vi "Omniax_mDrive_XYZR_2017APXNoBK.vi"() -> ()   [LabVIEW 2015]
uses:
  <vilib>/Utility/file.llb/Read From Spreadsheet File (I64).vi
  <vilib>/Utility/file.llb/Read From Spreadsheet File (string).vi
  <vilib>/Instr/_visa.llb/VISA Configure Serial Port (Instr).vi
  <vilib>/Utility/file.llb/Write To Spreadsheet File (I64).vi
  <vilib>/Utility/file.llb/Write To Spreadsheet File (string).vi
panel:
  out "Boolean 3":bool
  out "Boolean 2":bool
  out "Boolean":bool
  out "read buffer":string
  out "sum":dbl
  in  "Open?":bool
  out "Z max step":i32
  in  "V5 position 15360000":i32
  out "NC":bool
  out "R Velocity MVdeg/sec":dbl format="%.3f"
  out "R Position MV deg":dbl
  out "Z Velocity MV mm/sec":dbl format="%.3f"
  out "Z Position MV mm":dbl
  out "Y Velocity MV mm/sec":dbl format="%.3f"
  out "Y Position MV mm":dbl
  out "X Velocity MV mm/sec":dbl format="%.3f"
  out "X Position MV mm":dbl
  out "Presets":i32[][](array[numeric])
  in  "stop":bool
  in  "Tab Control 3":enum32{"Status", "Reset"}(tab)
  out "APX:Y_LIM":bool
  out "APX:MY_MVG":bool
  out "APX:X_LIM":bool
  out "APX:MX_MVG":bool
  out "APX:MZ_LIM":bool
  out "APX:MZ_MVG":bool
  out "APX:MR_LIM":bool
  out "APX:MR_MVG":bool
  out "APX:MX_RDY":bool
  out "APX:MY_RDY":bool
  out "APX:MZ_RDY":bool
  out "APX:MR_RDY":bool
  in  "Reset Y Position mm":dbl
  out "Reset Y Motor Steps":i32
  in  "Reset X Position mm":dbl
  out "Reset X Motor Steps":i32
  in  "Reset Z Position mm":dbl
  out "Reset Z Motor Steps":i32
  in  "Reset R Position deg":dbl
  out "Reset R Motor Steps":i32
  in  "Reset":bool
  in  "Tab Control":enum32{"mm", "preset", "step"}(tab)
  in  "APX:MX_RQ":dbl min=-1.28 max=1.28
  in  "APX:MX_VLC_RQ":dbl min=0.0 max=0.4 step=0.1
  in  "APX:MY_RQ":dbl min=-1.5 max=1.0
  in  "APX:MY_VLC_RQ":dbl min=0.0 max=0.4 step=0.1
  in  "APX:MZ_RQ":dbl=10.0 min=10.0 max=355.8 step=0.1
  in  "APX:MZ_VLC_RQ":dbl=0.20000000000000015 min=0.1 max=0.8 step=0.1
  in  "APX:MR_RQ":dbl
  in  "APX:MR_VLC_RQ":dbl
  in  "Add Button":bool
  in  "String":string
  in  "Delete Button":bool
  in  "Preset positions":i32(ring) items=["ZERO", "Default", "CDOSE", "QMS", "test", "test2", "test3", "yag position", "Sample Long Edge  ", "SPUTTER POS"]
  in  "Set Button":bool
  in  "X Velocity SP step/sec":i32 min=1 max=128000
  in  "Y Velocity SP step/sec":i32 min=1 max=128000
  in  "Z Velocity SP step/sec":i32 min=1 max=204800
  in  "R Velocity SP step/sec":i32 min=1 max=10000
  in  "Y Step SP":i32=-20000 min=-2304000 max=2304000 step=500
  in  "X Step SP":i32=-20000 min=-2304000 max=2304000 step=500
  in  "Z Step SP":i32=-20000 min=0 max=102400000 step=500
  in  "R Step SP":i32=-20000 min=-6144000 max=6144000 step=500
  out "X Step PV":i32 max=2000
  out "Y Step PV":i32 max=2000
  out "Z Step PV":i32 max=2000
  out "R Step PV":i32 max=2000
  in  "Clear ZY":bool
  out "R Backlash steps/sec":i32
  out "R Backlash":i32
  out "R Holding Current %":i32
  out "R Run Current %":i32
  out "R offset deg":dbl
  out "R deg/rev":dbl
  out "R steps/rev":u32
  out "R velocity PV step/sec":i32
  out "R MINPOS":i32=-94296
  out "R MAXPOS":i32=-34296
  out "R COM PORT":refnum<visa-resource-name>="COM5"
  out "APZ:MR_PV":dbl
  out "Z COM PORT":refnum<visa-resource-name>="COM5"
  out "Z Backlash steps/sec":i32
  out "Z Backlash":i32
  out "Z Holding Current %":i32
  out "Z Run Current %":i32
  out "Z offset mm":dbl
  out "Z mm/rev":dbl
  out "Z steps/rev":u32
  out "Z  velocity PV step/sec":i32
  out "Z MINPOS":i32=-94296
  out "Z MAXPOS":i32=-34296
  out "APX:MZ_PV":dbl
  out "APX:MX_PV":dbl
  out "X velocity PV step/sec":i32
  out "X Backlash steps/sec":i32
  out "X Backlash":i32
  out "X Holding Current %":i32
  out "X Run Current %":i32
  out "X offset mm":dbl
  out "X mm/rev":dbl
  out "X steps/rev":u32
  out "X MAXPOS":i32=-34296
  out "X MINPOS":i32=-94296
  out "X COM PORT":refnum<visa-resource-name>="COM5"
  out "Y Backlash steps/sec":i32
  out "Y Backlash":i32
  out "Y Holding Current %":i32
  out "Y Run Current %":i32
  out "APX:MY_PV":dbl
  out "Y offset mm":dbl
  out "Y mm/rev":dbl
  out "Y steps/rev":u32
  out "Y velocity PV step/sec":i32
  in  "APX:MXYZR_STOP":bool
  out "Y MINPOS":i32=-94296
  out "Y MAXPOS":i32=-34296
  out "Y COM PORT":refnum<visa-resource-name>="COM5"
  # "12-15"
  # "Current position"
  # "Goto position"
  # "MX"
  # "MY"
  # "MZ"
  # "MR"
  # "Preset position"
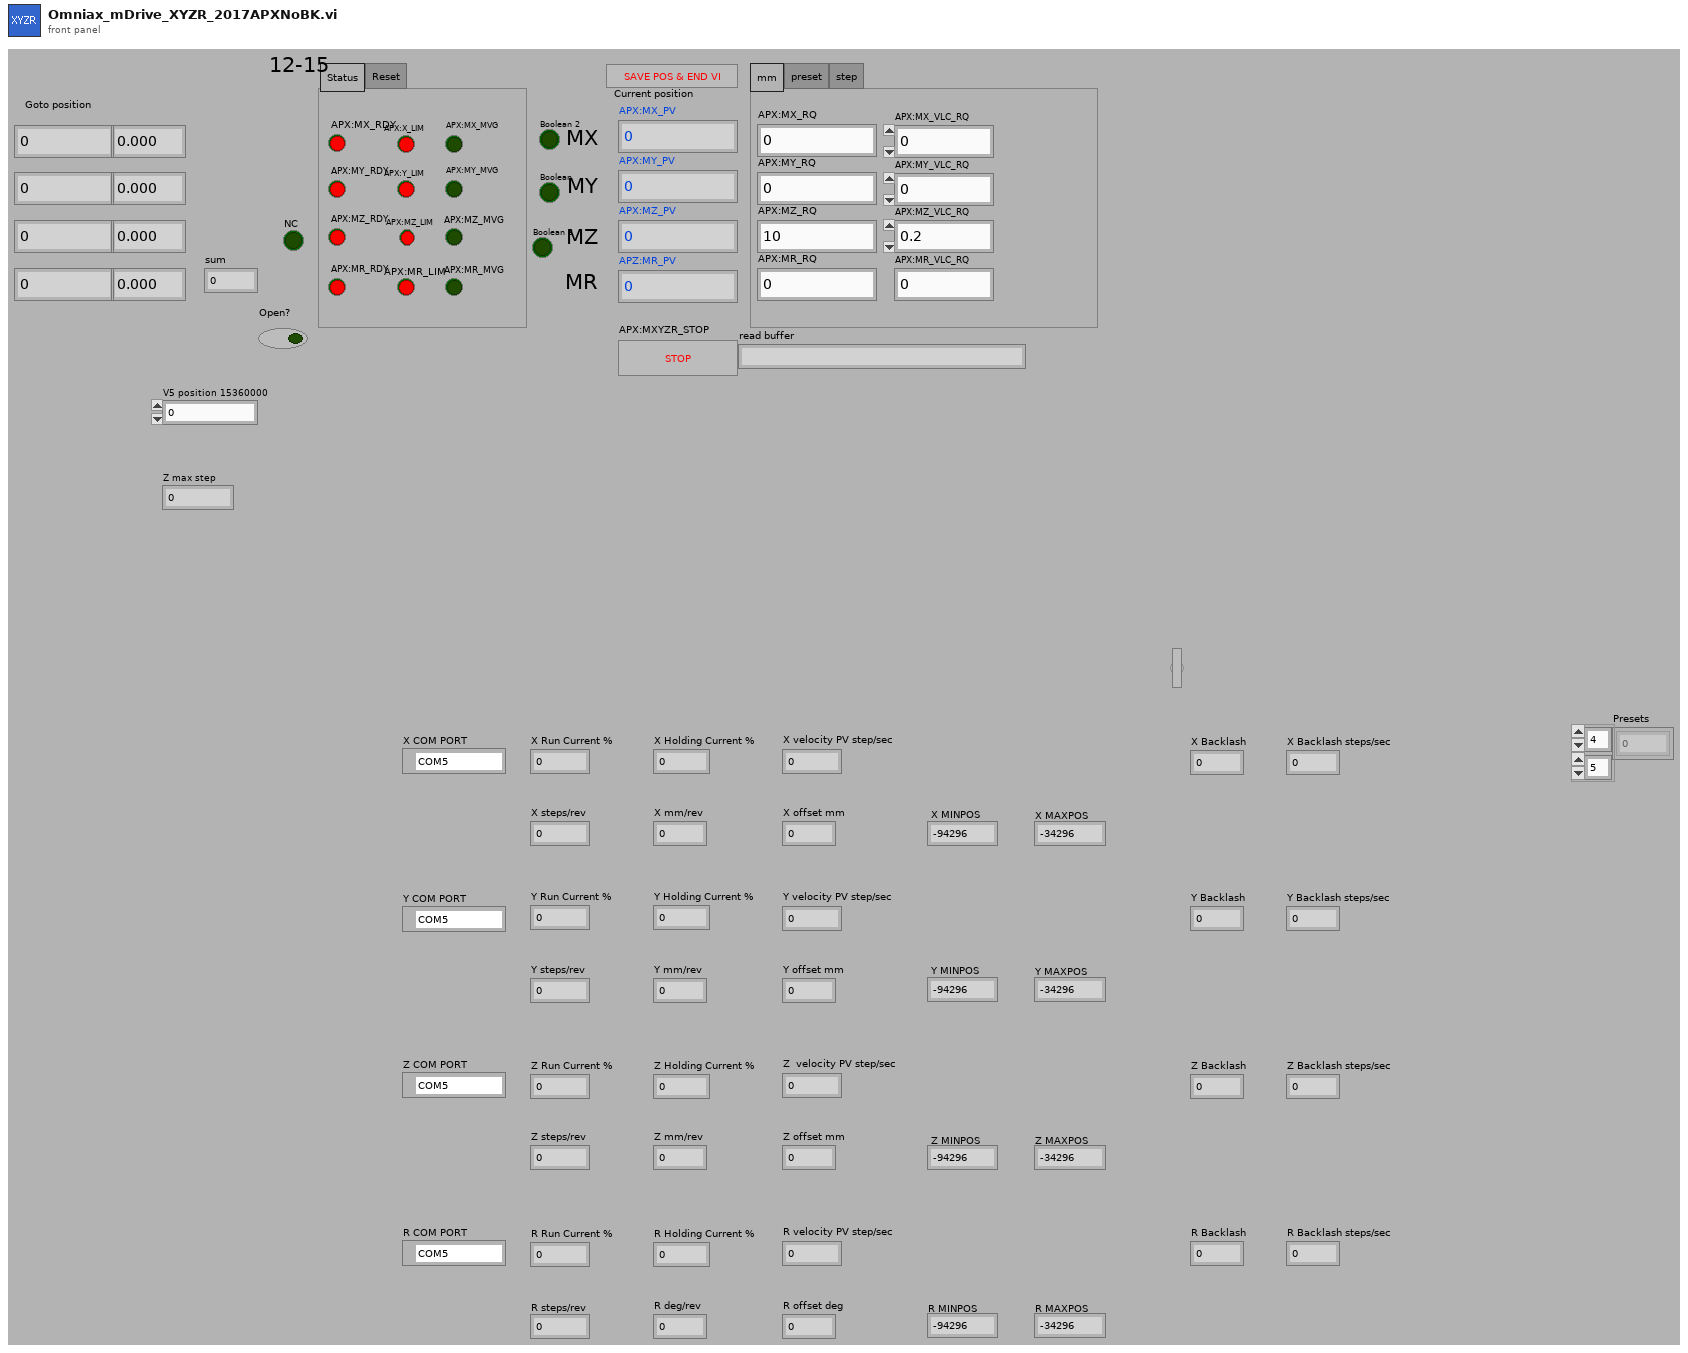
[diagram p1: front panel]
types:
  T1 = enum16{"Stop", "Reset", "Run Current", "Holding Current", "Accel Rate", "Decel Rate", "Move to Relative Position", "Move to Absolute Position", "Echo Mode", "Print Parameter", "Send String", "Microstep Resolution", "Set Current Position", "Max Velocity"}
  T2 = enum8{"Enabled", "Disabled", "Disabled and Grayed Out"}
  T3 = cluster{"first row[0]":i64, "first row[1]":i64, "first row[2]":i64, "first row[3]":i64, "first row[4]":i64, "first row[5]":i64, "first row[6]":i64, "first row[7]":i64, "first row[8]":i64}
  T4 = cluster{"Value[0]":i32, "Value[1]":i32, "Value[2]":i32, "Value[3]":i32, "Value[4]":i32, "Value[5]":i32, "Value[6]":i32, "Value[7]":i32, "Value[8]":i32}
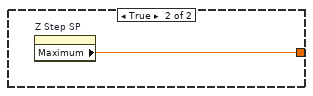
[diagram p9: hidden frame]
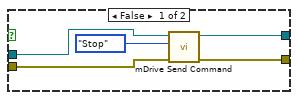
[diagram p15: hidden frame]
diagram:
  w2 = 0 ("dimension size")
  n1 = disable-structure shown="Disabled" {
    disable-tunnel: [w106 _] -> _
    disable-tunnel: [w105 _] -> _
    frame Disabled {
      n2 = call "DigitalIO_sub_V5_MON.vi"() -> ("CL"=w105:bool, "OP"=w106:bool)  [unwired: 8 in]
    }
    frame Enabled {
    }
  }
  n3 = disable-structure shown="Disabled" {
    frame Disabled {
      n4 = flat-sequence {
        frame #0 {
          w107 = FALSE ("Value (Signaling)")
          w110 = FALSE ("Value (Signaling)")
          w113 = FALSE ("Value (Signaling)")
          w114 = FALSE ("Value (Signaling)")
          "Z Backlash steps/sec" <- 25600 ("Z Backlash steps/sec")
          "Z Backlash" <- -51200 ("Z Backlash")
          "X Backlash steps/sec" <- 25600 ("Value (Signaling)")
          "X Backlash" <- 10240 ("Backlash2")
          "Y Backlash" <- -10240 ("Backlash2")
          "Y Backlash steps/sec" <- 25600 ("Value (Signaling)")
          "R Backlash steps/sec" <- 6400 ("R Backlash steps/sec")
          "R Backlash" <- -12800 ("R Backlash")
        }
      }
    }
    frame Enabled {
    }
  }
  n5 = flat-sequence {
    tunnel: [w120] -> w34
    tunnel: [w119] -> w33
    tunnel: [w132] -> w50
    tunnel: [w130] -> w48
    tunnel: w34 -> [w129]
    tunnel: w33 -> [w131]
    tunnel: w50 -> [w138]
    tunnel: [w139] -> w49
    tunnel: w48 -> [w135]
    tunnel: [w137] -> w47
    tunnel: [w148] -> w100
    tunnel: [w150] -> w98
    tunnel: w49 -> [w149]
    tunnel: w47 -> [w151]
    tunnel: w100 -> [w158]
    tunnel: [w157] -> w99
    tunnel: w98 -> [w155]
    tunnel: [w156] -> w97
    tunnel: [w168] -> w102
    tunnel: [w169] -> w101
    tunnel: w99 -> [w167]
    tunnel: w97 -> [w166]
    tunnel: w102 -> [w179]
    tunnel: w101 -> [w178]
    tunnel: [w181] -> w86
    tunnel: [w180] -> w85
    tunnel: [w175] -> w84
    tunnel: [w186] -> w103
    tunnel: [w187] -> w104
    tunnel: w86 -> [w187]
    tunnel: w85 -> [w186]
    tunnel: w84 -> [w182]
    frame #0 {
      w127 = refnum<visa-resource-name> "COM13" ("COM PORT")
      w125 = u16 0 items=["None", "XON/XOFF", "RTS/CTS", "XON/XOFF & RTS/CTS", "DTR/DSR", "XON/XOFF & DTR/DSR"] ("flow control (0:none)")
      w124 = u16 10 items=["1.0"=10, "1.5"=15, "2.0"=20] ("stop bits (10: 1 bit)")
      # "Stop bits"
      n6 = call-poly "VISA Configure Serial Port"("VISA resource name"=w127, "timeout (10sec)"=u32 10000, "baud rate (9600)"=u32 9600, "data bits (8)"=u16 8, "parity (0:none)"=enum16{"None", "Odd", "Even", "Mark", "Space"}."None", "stop bits (10: 1 bit)"=w124, "flow control (0:none)"=w125) -> ("VISA resource name out"=w120:refnum<visa-resource-name>, "error out"=w119:errorcluster)  [unwired: 7 in]
      "Y COM PORT" <- w127
    }
    frame #1 {
      n7 = VISA Flush I/O Buffer(VISA resource name=w129) -> (VISA resource name out=w128:refnum<visa-resource-name>)  [unwired: 2 in, 1 out]
      n8 = call "mDrive Send Command.vi"("error in (no error)"=w131, "Extra"="EM 2", "Command"=T1."Send String", "VISA resource name"=w128) -> ("error out"=w130:errorcluster, "VISA resource name out"=w132:refnum<visa-resource-name>)  [unwired: 3 in, 1 out]
    }
    frame #2 {
      n9 = Number To Decimal String(number=1000000) -> (decimal integer string=w140:string)  [unwired: 1 in]
      n10 = call "mDrive Send Command.vi"("error in (no error)"=w135, "Extra"=w140, "Command"=T1."Accel Rate", "VISA resource name"=w138) -> ("error out"=w136:errorcluster, "VISA resource name out"=w144:refnum<visa-resource-name>)  [unwired: 3 in, 1 out]
      n11 = call "mDrive Send Command.vi"("error in (no error)"=w136, "Extra"=w140, "Command"=T1."Decel Rate", "VISA resource name"=w144) -> ("error out"=w137:errorcluster, "VISA resource name out"=w139:refnum<visa-resource-name>)  [unwired: 3 in, 1 out]
    }
    frame #3 {
      # "Run Current %"
      n12 = property on="Y Run Current %" class="DigNum (strict)"() -> ("Value"=w146:i32)  [unwired: 2 in, 2 out]
      n13 = Number To Decimal String(number=w146) -> (decimal integer string=w147:string)  [unwired: 1 in]
      n14 = call "mDrive Send Command.vi"("error in (no error)"=w151, "Extra"=w147, "Command"=T1."Run Current", "VISA resource name"=w149) -> ("error out"=w150:errorcluster, "VISA resource name out"=w148:refnum<visa-resource-name>)  [unwired: 3 in, 1 out]
    }
    frame #4 {
      # "Holding Current %"
      n15 = property on="Y Holding Current %" class="DigNum (strict)"() -> ("Value"=w153:i32)  [unwired: 2 in, 2 out]
      n16 = Number To Decimal String(number=w153) -> (decimal integer string=w154:string)  [unwired: 1 in]
      n17 = call "mDrive Send Command.vi"("error in (no error)"=w155, "Extra"=w154, "Command"=T1."Holding Current", "VISA resource name"=w158) -> ("error out"=w156:errorcluster, "VISA resource name out"=w157:refnum<visa-resource-name>)  [unwired: 3 in, 1 out]
    }
    frame #5 {
      # "Velocity Max"
      n18 = property on="Y Velocity SP step/sec" class="DigNum (strict)"() -> ("Value"=w165:i32)  [unwired: 2 in, 2 out]
      n19 = Number To Decimal String(number=w165) -> (decimal integer string=w164:string)  [unwired: 1 in]
      n20 = call "mDrive Send Command.vi"("error in (no error)"=w166, "Extra"=w164, "Command"=T1."Max Velocity", "VISA resource name"=w167) -> ("error out"=w162:errorcluster, "VISA resource name out"=w172:refnum<visa-resource-name>)  [unwired: 3 in, 1 out]
      n21 = call "mDrive Send Command.vi"("error in (no error)"=w162, "Extra"="VM", "Command"=T1."Print Parameter", "VISA resource name"=w172) -> ("error out"=w169:errorcluster, "read buffer"=w170:string, "VISA resource name out"=w168:refnum<visa-resource-name>)  [unwired: 3 in]
      n22 = Decimal String To Number(string=w170, offset=0) -> (number=w163:i32)  [unwired: 1 in, 1 out]
      n23 = property on="Y scan velocity MV step/sec" class="DigNum (strict)"("Val(Sgnl)"=w163) -> ()  [unwired: 2 in, 2 out]
    }
    frame #6 {
      # "PRINT POSITION"
      n24 = call "mDrive Send Command.vi"("error in (no error)"=w178, "Extra"="P", "Command"=T1."Print Parameter", "VISA resource name"=w179) -> ("error out"=w180:errorcluster, "read buffer"=w177:string, "VISA resource name out"=w181:refnum<visa-resource-name>)  [unwired: 3 in]
      n25 = Decimal String To Number(string=w177, offset=0) -> (number=w175:i32)  [unwired: 1 in, 1 out]
    }
    frame #7 {
      w184 = -2304000 ("lower limit")
      w185 = 2304000 ("upper limit")
      n26 = property on="Y Step SP" class="DigNum (strict)"("Val(Sgnl)"=w182) -> ()  [unwired: 2 in, 2 out]
      n27 = property on="Y Step SP" class="DigNum (strict)"("Maximum"=w185) -> ()  [unwired: 2 in, 2 out]
      n28 = In Range and Coerce(upper limit=w185, x=w182, lower limit=w184) -> (In Range?=w183:bool)  [unwired: 1 out]
      n29 = property on="Y Step SP" class="DigNum (strict)"("Minimum"=w184) -> ()  [unwired: 2 in, 2 out]
      n30 = property on="APX:Y_LIM" class="Bool (strict)"("Val(Sgnl)"=w183) -> ()  [unwired: 2 in, 2 out]
      "Y MINPOS" <- w184
      "Y MAXPOS" <- w185
    }
  }
  n31 = flat-sequence {
    tunnel: [w189] -> w36
    tunnel: [w188] -> w35
    tunnel: [w197] -> w54
    tunnel: [w199] -> w52
    tunnel: w36 -> [w198]
    tunnel: w35 -> [w200]
    tunnel: w54 -> [w204]
    tunnel: [w205] -> w53
    tunnel: w52 -> [w203]
    tunnel: [w206] -> w51
    tunnel: [w217] -> w71
    tunnel: [w219] -> w70
    tunnel: w53 -> [w218]
    tunnel: w51 -> [w213]
    tunnel: w71 -> [w226]
    tunnel: [w225] -> w69
    tunnel: w70 -> [w223]
    tunnel: [w224] -> w68
    tunnel: [w236] -> w67
    tunnel: [w237] -> w66
    tunnel: w69 -> [w235]
    tunnel: w68 -> [w234]
    tunnel: w67 -> [w247]
    tunnel: w66 -> [w246]
    tunnel: [w249] -> w65
    tunnel: [w248] -> w64
    tunnel: [w243] -> w63
    tunnel: [w256] -> w59
    tunnel: [w257] -> w60
    tunnel: w65 -> [w257]
    tunnel: w64 -> [w256]
    tunnel: w63 -> [w254]
    frame #0 {
      w196 = refnum<visa-resource-name> "COM15" ("COM PORT")
      w194 = u16 0 items=["None", "XON/XOFF", "RTS/CTS", "XON/XOFF & RTS/CTS", "DTR/DSR", "XON/XOFF & DTR/DSR"] ("flow control (0:none)")
      w193 = u16 10 items=["1.0"=10, "1.5"=15, "2.0"=20] ("stop bits (10: 1 bit)")
      # "Stop bits"
      n32 = call-poly "VISA Configure Serial Port"("VISA resource name"=w196, "timeout (10sec)"=u32 10000, "baud rate (9600)"=u32 9600, "data bits (8)"=u16 8, "parity (0:none)"=enum16{"None", "Odd", "Even", "Mark", "Space"}."None", "stop bits (10: 1 bit)"=w193, "flow control (0:none)"=w194) -> ("VISA resource name out"=w189:refnum<visa-resource-name>, "error out"=w188:errorcluster)  [unwired: 7 in]
      "R COM PORT" <- w196
    }
    frame #1 {
      n33 = call "mDrive Send Command.vi"("error in (no error)"=w200, "Extra"="EM 2", "Command"=T1."Send String", "VISA resource name"=w198) -> ("error out"=w199:errorcluster, "VISA resource name out"=w197:refnum<visa-resource-name>)  [unwired: 3 in, 1 out]
    }
    frame #2 {
      # "pr=1000000"
      n34 = Number To Decimal String(number=100000) -> (decimal integer string=w208:string)  [unwired: 1 in]
      n35 = call "mDrive Send Command.vi"("error in (no error)"=w203, "Extra"=w208, "Command"=T1."Accel Rate", "VISA resource name"=w204) -> ("error out"=w207:errorcluster, "VISA resource name out"=w212:refnum<visa-resource-name>)  [unwired: 3 in, 1 out]
      n36 = call "mDrive Send Command.vi"("error in (no error)"=w207, "Extra"=w208, "Command"=T1."Decel Rate", "VISA resource name"=w212) -> ("error out"=w206:errorcluster, "VISA resource name out"=w205:refnum<visa-resource-name>)  [unwired: 3 in, 1 out]
    }
    frame #3 {
      # "Run Current %"
      n37 = property on="R Run Current %" class="DigNum (strict)"() -> ("Value"=w215:i32)  [unwired: 2 in, 2 out]
      n38 = Number To Decimal String(number=w215) -> (decimal integer string=w216:string)  [unwired: 1 in]
      n39 = call "mDrive Send Command.vi"("error in (no error)"=w213, "Extra"=w216, "Command"=T1."Run Current", "VISA resource name"=w218) -> ("error out"=w219:errorcluster, "VISA resource name out"=w217:refnum<visa-resource-name>)  [unwired: 3 in, 1 out]
    }
    frame #4 {
      # "Holding Current %"
      n40 = property on="R Holding Current %" class="DigNum (strict)"() -> ("Value"=w221:i32)  [unwired: 2 in, 2 out]
      n41 = Number To Decimal String(number=w221) -> (decimal integer string=w222:string)  [unwired: 1 in]
      n42 = call "mDrive Send Command.vi"("error in (no error)"=w223, "Extra"=w222, "Command"=T1."Holding Current", "VISA resource name"=w226) -> ("error out"=w224:errorcluster, "VISA resource name out"=w225:refnum<visa-resource-name>)  [unwired: 3 in, 1 out]
    }
    frame #5 {
      # "Print Velocity Max"
      # "Velocity Max"
      n43 = property on="R Velocity SP step/sec" class="DigNum (strict)"() -> ("Value"=w233:i32)  [unwired: 2 in, 2 out]
      n44 = Number To Decimal String(number=w233) -> (decimal integer string=w232:string)  [unwired: 1 in]
      n45 = call "mDrive Send Command.vi"("error in (no error)"=w234, "Extra"=w232, "Command"=T1."Max Velocity", "VISA resource name"=w235) -> ("error out"=w230:errorcluster, "VISA resource name out"=w240:refnum<visa-resource-name>)  [unwired: 3 in, 1 out]
      n46 = call "mDrive Send Command.vi"("error in (no error)"=w230, "Extra"="VM", "Command"=T1."Print Parameter", "VISA resource name"=w240) -> ("error out"=w237:errorcluster, "read buffer"=w238:string, "VISA resource name out"=w236:refnum<visa-resource-name>)  [unwired: 3 in]
      n47 = Decimal String To Number(string=w238, offset=0) -> (number=w231:i32)  [unwired: 1 in, 1 out]
      n48 = property on="R velocity PV step/sec" class="DigNum (strict)"("Val(Sgnl)"=w231) -> ()  [unwired: 2 in, 2 out]
    }
    frame #6 {
      # "PRINT POSITION"
      n49 = call "mDrive Send Command.vi"("error in (no error)"=w246, "Extra"="P", "Command"=T1."Print Parameter", "VISA resource name"=w247) -> ("error out"=w248:errorcluster, "read buffer"=w245:string, "VISA resource name out"=w249:refnum<visa-resource-name>)  [unwired: 3 in]
      n50 = Decimal String To Number(string=w245, offset=0) -> (number=w243:i32)  [unwired: 1 in, 1 out]
    }
    frame #7 {
      n51 = property on="R Step SP" class="DigNum (strict)"("Val(Sgnl)"=w254) -> ()  [unwired: 2 in, 2 out]
      n52 = property on="R Step SP" class="DigNum (strict)"() -> ("Maximum"=w253:dbl)  [unwired: 2 in, 2 out]
      n53 = property on="R Step SP" class="DigNum (strict)"() -> ("Minimum"=w252:dbl)  [unwired: 2 in, 2 out]
      n54 = To Long Integer(number=w253) -> (32bit integer=w250:i32)
      "R MAXPOS" <- w250
      n55 = To Long Integer(number=w252) -> (32bit integer=w251:i32)
      "R MINPOS" <- w251
      n56 = In Range and Coerce(upper limit=w250, x=w254, lower limit=w251) -> (In Range?=w255:bool)  [unwired: 1 out]
      n57 = property on="APX:MR_LIM" class="Bool (strict)"("Val(Sgnl)"=w255) -> ()  [unwired: 2 in, 2 out]
    }
  }
  n58 = flat-sequence {
    frame #0 {
      w263 = -3.0 ("R deg/rev")
      w261 = u32 51200 ("step/rev")
      w265 = 10000 ("Value (Signaling)")
      n59 = To Double Precision Float(number=w265) -> (double precision float=w267:dbl)
      n60 = To Double Precision Float(number=w261) -> (double precision float=w262:dbl)
      n61 = property on="R Velocity SP step/sec" class="DigNum (strict)"("Val(Sgnl)"=w265) -> ()  [unwired: 2 in, 2 out]
      n62 = property on="R Velocity SP step/sec" class="DigNum (strict)"("Minimum"=1.0 ("Data Entry Limits:Minimum")) -> ()  [unwired: 2 in, 2 out]
      n63 = Divide(x=w267, y=w262) -> (x/y=w266:dbl)
      n64 = property on="R Velocity SP step/sec" class="DigNum (strict)"("Maximum"=w267) -> ()  [unwired: 2 in, 2 out]
      n65 = Multiply(x=w266, y=w263) -> (x*y=w264:dbl)
      n66 = Absolute Value(x=w264) -> (abs(x)=w258:dbl)
      n67 = property on="APX:MR_VLC_RQ" class="DigNum (strict)"("Val(Sgnl)"=w258) -> ()  [unwired: 2 in, 2 out]
      "R offset deg" <- 0.0 ("R offset deg")
      "R deg/rev" <- w263
      "R steps/rev" <- w261
    }
  }
  n68 = flat-sequence {
    frame #0 {
      w269 = 0.2 ("Z mm/rev")
      w268 = u32 51200 ("step/rev")
      w270 = 204800 ("Value (Signaling)")
      n69 = To Double Precision Float(number=w270) -> (double precision float=w274:dbl)
      n70 = To Double Precision Float(number=w268) -> (double precision float=w273:dbl)
      n71 = property on="Z Velocity SP step/sec" class="DigNum (strict)"("Val(Sgnl)"=w270) -> ()  [unwired: 2 in, 2 out]
      n72 = property on="Z Velocity SP step/sec" class="DigNum (strict)"("Minimum"=1.0 ("Data Entry Limits:Minimum")) -> ()  [unwired: 2 in, 2 out]
      n73 = Divide(x=w274, y=w273) -> (x/y=w271:dbl)
      n74 = property on="Z Velocity SP step/sec" class="DigNum (strict)"("Maximum"=w274) -> ()  [unwired: 2 in, 2 out]
      n75 = Multiply(x=w271, y=w269) -> (x*y=w272:dbl)
      n76 = property on="APX:MZ_VLC_RQ" class="DigNum (strict)"("Val(Sgnl)"=w272) -> ()  [unwired: 2 in, 2 out]
      "Z offset mm" <- 0.0 ("Z offset mm")
      "Z mm/rev" <- w269
      "Z steps/rev" <- w268
    }
  }
  n77 = flat-sequence {
    frame #0 {
      "Z Holding Current %" <- 20 ("Z Holding Current %")
      "Z Run Current %" <- 40 ("Z Run Current %")
      "X Run Current %" <- 40 ("Run Current %")
      "X Holding Current %" <- 20 ("Holding Current %")
      "Y Run Current %" <- 40 ("Run Current %")
      "Y Holding Current %" <- 20 ("Holding Current %")
      "R Holding Current %" <- 15 ("R Holding Current %")
      "R Run Current %" <- 80 ("R Run Current %")
    }
  }
  n78 = flat-sequence {
    frame #0 {
      (unwired) FALSE ("Value (Signaling)")
      (unwired) T2."Disabled and Grayed Out" ("Disabled")
      (unwired) T2."Disabled and Grayed Out" ("Disabled")
      (unwired) 0.1 ("Value (Signaling)")
      (unwired) FALSE ("Value (Signaling)")
      (unwired) 0.1 ("Value (Signaling)")
      (unwired) FALSE ("Value (Signaling)")
      (unwired) 0.1 ("Value (Signaling)")
      (unwired) FALSE ("Value (Signaling)")
      n79 = property on="APX:MR_VLC_RQ" class="DigNum (strict)"("Val(Sgnl)"=0.1 ("Value (Signaling)")) -> ()  [unwired: 2 in, 2 out]
    }
  }
  n80 = flat-sequence {
    frame #0 {
      w288 = 0.2 ("MM/rev")
      w291 = u32 51200 ("step/rev")
      w286 = 128000 ("Value (Signaling)")
      # "a=1000000"
      n81 = property on="X Velocity SP step/sec" class="DigNum (strict)"("Minimum"=1.0 ("Data Entry Limits:Minimum")) -> ()  [unwired: 2 in, 2 out]
      n82 = To Double Precision Float(number=w286) -> (double precision float=w292:dbl)
      n83 = To Double Precision Float(number=w291) -> (double precision float=w290:dbl)
      n84 = property on="X Velocity SP step/sec" class="DigNum (strict)"("Val(Sgnl)"=w286) -> ()  [unwired: 2 in, 2 out]
      n85 = property on="X Velocity SP step/sec" class="DigNum (strict)"("Maximum"=w292) -> ()  [unwired: 2 in, 2 out]
      n86 = Divide(x=w292, y=w290) -> (x/y=w287:dbl)
      n87 = Multiply(x=w287, y=w288) -> (x*y=w289:dbl)
      n88 = property on="APX:MX_VLC_RQ" class="DigNum (strict)"("Val(Sgnl)"=w289) -> ()  [unwired: 2 in, 2 out]
      "X offset mm" <- 0.0 ("offset")
      "X steps/rev" <- w291
      "X mm/rev" <- w288
    }
  }
  n89 = flat-sequence {
    frame #0 {
      w297 = 0.2 ("MM/rev")
      w300 = u32 51200 ("step/rev")
      w295 = 128000 ("Value (Signaling)")
      n90 = To Double Precision Float(number=w295) -> (double precision float=w301:dbl)
      n91 = To Double Precision Float(number=w300) -> (double precision float=w299:dbl)
      n92 = property on="Y Velocity SP step/sec" class="DigNum (strict)"("Val(Sgnl)"=w295) -> ()  [unwired: 2 in, 2 out]
      n93 = property on="Y Velocity SP step/sec" class="DigNum (strict)"("Minimum"=1.0 ("Data Entry Limits:Minimum")) -> ()  [unwired: 2 in, 2 out]
      n94 = Divide(x=w301, y=w299) -> (x/y=w296:dbl)
      n95 = property on="Y Velocity SP step/sec" class="DigNum (strict)"("Maximum"=w301) -> ()  [unwired: 2 in, 2 out]
      n96 = Multiply(x=w296, y=w297) -> (x*y=w298:dbl)
      n97 = property on="APX:MY_VLC_RQ" class="DigNum (strict)"("Val(Sgnl)"=w298) -> ()  [unwired: 2 in, 2 out]
      "Y offset mm" <- 0.0 ("offset")
      "Y steps/rev" <- w300
      "Y mm/rev" <- w297
    }
  }
  n98 = property on="Z Step SP" class="DigNum (strict)"("Minimum"=0 ("lower limit")) -> ()  [unwired: 2 in, 2 out]
  n99 = flat-sequence {
    tunnel: [w304] -> w40
    tunnel: [w305] -> w39
    tunnel: [w315] -> w46
    tunnel: [w314] -> w44
    tunnel: w40 -> [w316]
    tunnel: w39 -> [w313]
    tunnel: w46 -> [w326]
    tunnel: [w321] -> w45
    tunnel: w44 -> [w325]
    tunnel: [w325] -> w43
    tunnel: [w330] -> w80
    tunnel: [w332] -> w79
    tunnel: w45 -> [w331]
    tunnel: w43 -> [w333]
    tunnel: w80 -> [w340]
    tunnel: [w339] -> w78
    tunnel: w79 -> [w337]
    tunnel: [w338] -> w77
    tunnel: [w350] -> w76
    tunnel: [w351] -> w75
    tunnel: w78 -> [w349]
    tunnel: w77 -> [w348]
    tunnel: w76 -> [w361]
    tunnel: w75 -> [w360]
    tunnel: [w363] -> w74
    tunnel: [w362] -> w73
    tunnel: [w357] -> w72
    tunnel: [w370] -> w61
    tunnel: [w371] -> w62
    tunnel: w74 -> [w371]
    tunnel: w73 -> [w370]
    tunnel: w72 -> [w368]
    frame #0 {
      w312 = refnum<visa-resource-name> "COM14" ("COM PORT")
      w310 = u16 0 items=["None", "XON/XOFF", "RTS/CTS", "XON/XOFF & RTS/CTS", "DTR/DSR", "XON/XOFF & DTR/DSR"] ("flow control (0:none)")
      w309 = u16 10 items=["1.0"=10, "1.5"=15, "2.0"=20] ("stop bits (10: 1 bit)")
      # "Stop bits"
      n100 = call-poly "VISA Configure Serial Port"("VISA resource name"=w312, "timeout (10sec)"=u32 10000, "baud rate (9600)"=u32 9600, "data bits (8)"=u16 8, "parity (0:none)"=enum16{"None", "Odd", "Even", "Mark", "Space"}."None", "stop bits (10: 1 bit)"=w309, "flow control (0:none)"=w310) -> ("VISA resource name out"=w304:refnum<visa-resource-name>, "error out"=w305:errorcluster)  [unwired: 7 in]
      "Z COM PORT" <- w312
    }
    frame #1 {
      n101 = call "mDrive Send Command.vi"("error in (no error)"=w313, "Extra"="EM 2", "Command"=T1."Send String", "VISA resource name"=w316) -> ("error out"=w314:errorcluster, "VISA resource name out"=w315:refnum<visa-resource-name>)  [unwired: 3 in, 1 out]
    }
    frame #2 {
      n102 = Number To Decimal String(number=1000000) -> (decimal integer string=w319:string)  [unwired: 1 in]
      n103 = call "mDrive Send Command.vi"("Extra"=w319, "Command"=T1."Accel Rate", "VISA resource name"=w326) -> ("VISA resource name out"=w324:refnum<visa-resource-name>)  [unwired: 4 in, 2 out]
      n104 = call "mDrive Send Command.vi"("Extra"=w319, "Command"=T1."Decel Rate", "VISA resource name"=w324) -> ("VISA resource name out"=w321:refnum<visa-resource-name>)  [unwired: 4 in, 2 out]
    }
    frame #3 {
      # "Run Current %"
      n105 = property on="Z Run Current %" class="DigNum (strict)"() -> ("Value"=w328:i32)  [unwired: 2 in, 2 out]
      n106 = Number To Decimal String(number=w328) -> (decimal integer string=w329:string)  [unwired: 1 in]
      n107 = call "mDrive Send Command.vi"("error in (no error)"=w333, "Extra"=w329, "Command"=T1."Run Current", "VISA resource name"=w331) -> ("error out"=w332:errorcluster, "VISA resource name out"=w330:refnum<visa-resource-name>)  [unwired: 3 in, 1 out]
    }
    frame #4 {
      # "Holding Current %"
      n108 = property on="Z Run Current %" class="DigNum (strict)"() -> ("Value"=w335:i32)  [unwired: 2 in, 2 out]
      n109 = Number To Decimal String(number=w335) -> (decimal integer string=w336:string)  [unwired: 1 in]
      n110 = call "mDrive Send Command.vi"("error in (no error)"=w337, "Extra"=w336, "Command"=T1."Holding Current", "VISA resource name"=w340) -> ("error out"=w338:errorcluster, "VISA resource name out"=w339:refnum<visa-resource-name>)  [unwired: 3 in, 1 out]
    }
    frame #5 {
      # "Velocity Max"
      n111 = property on="Z Velocity SP step/sec" class="DigNum (strict)"() -> ("Value"=w347:i32)  [unwired: 2 in, 2 out]
      n112 = Number To Decimal String(number=w347) -> (decimal integer string=w346:string)  [unwired: 1 in]
      n113 = call "mDrive Send Command.vi"("error in (no error)"=w348, "Extra"=w346, "Command"=T1."Max Velocity", "VISA resource name"=w349) -> ("error out"=w344:errorcluster, "VISA resource name out"=w354:refnum<visa-resource-name>)  [unwired: 3 in, 1 out]
      n114 = call "mDrive Send Command.vi"("error in (no error)"=w344, "Extra"="VM", "Command"=T1."Print Parameter", "VISA resource name"=w354) -> ("error out"=w351:errorcluster, "read buffer"=w352:string, "VISA resource name out"=w350:refnum<visa-resource-name>)  [unwired: 3 in]
      n115 = Decimal String To Number(string=w352, offset=0) -> (number=w345:i32)  [unwired: 1 in, 1 out]
      n116 = property on="Z  velocity PV step/sec" class="DigNum (strict)"("Val(Sgnl)"=w345) -> ()  [unwired: 2 in, 2 out]
    }
    frame #6 {
      # "PRINT POSITION"
      n117 = call "mDrive Send Command.vi"("error in (no error)"=w360, "Extra"="P", "Command"=T1."Print Parameter", "VISA resource name"=w361) -> ("error out"=w362:errorcluster, "read buffer"=w359:string, "VISA resource name out"=w363:refnum<visa-resource-name>)  [unwired: 3 in]
      n118 = Decimal String To Number(string=w359, offset=0) -> (number=w357:i32)  [unwired: 1 in, 1 out]
    }
    frame #7 {
      n119 = property on="Z Step SP" class="DigNum (strict)"("Val(Sgnl)"=w368) -> ()  [unwired: 2 in, 2 out]
      n120 = property on="Z Step SP" class="DigNum (strict)"() -> ("Maximum"=w365:dbl)  [unwired: 2 in, 2 out]
      n121 = property on="Z Step SP" class="DigNum (strict)"() -> ("Minimum"=w367:dbl)  [unwired: 2 in, 2 out]
      n122 = To Long Integer(number=w365) -> (32bit integer=w366:i32)
      "Z MAXPOS" <- w366
      n123 = To Long Integer(number=w367) -> (32bit integer=w364:i32)
      "Z MINPOS" <- w364
      n124 = In Range and Coerce(upper limit=w366, x=w368, lower limit=w364) -> (In Range?=w369:bool)  [unwired: 1 out]
      n125 = property on="APX:MZ_LIM" class="Bool (strict)"("Val(Sgnl)"=w369) -> ()  [unwired: 2 in, 2 out]
    }
  }
  n126 = property on="R Step SP" class="DigNum (strict)"("Maximum"=6144000 ("upper limit")) -> ()  [unwired: 2 in, 2 out]
  n127 = property on="R Step SP" class="DigNum (strict)"("Minimum"=-6144000 ("lower limit")) -> ()  [unwired: 2 in, 2 out]
  n128 = property on="V5 position 15360000" class="DigNum (strict)"("Value"=15360000 ("V5 position 15360000")) -> ()  [unwired: 2 in, 2 out]
  n129 = property on="Z Step SP" class="DigNum (strict)"("Maximum"=102400000 ("upper limit")) -> ()  [unwired: 2 in, 2 out]
  n130 = flat-sequence {
    tunnel: [w373] -> w38
    tunnel: [w372] -> w37
    tunnel: [w385] -> w58
    tunnel: [w383] -> w56
    tunnel: w38 -> [w382]
    tunnel: w37 -> [w384]
    tunnel: w58 -> [w389]
    tunnel: [w388] -> w57
    tunnel: w56 -> [w390]
    tunnel: [w392] -> w55
    tunnel: [w401] -> w96
    tunnel: [w403] -> w95
    tunnel: w57 -> [w402]
    tunnel: w55 -> [w404]
    tunnel: w96 -> [w411]
    tunnel: [w410] -> w94
    tunnel: w95 -> [w408]
    tunnel: [w409] -> w93
    tunnel: [w421] -> w92
    tunnel: [w422] -> w91
    tunnel: w94 -> [w420]
    tunnel: w93 -> [w419]
    tunnel: w92 -> [w432]
    tunnel: w91 -> [w431]
    tunnel: [w434] -> w83
    tunnel: [w433] -> w82
    tunnel: [w428] -> w81
    tunnel: [w439] -> w89
    tunnel: [w440] -> w90
    tunnel: w83 -> [w440]
    tunnel: w82 -> [w439]
    tunnel: w81 -> [w435]
    frame #0 {
      w380 = refnum<visa-resource-name> "COM12" ("COM PORT")
      w378 = u16 0 items=["None", "XON/XOFF", "RTS/CTS", "XON/XOFF & RTS/CTS", "DTR/DSR", "XON/XOFF & DTR/DSR"] ("flow control (0:none)")
      w377 = u16 10 items=["1.0"=10, "1.5"=15, "2.0"=20] ("stop bits (10: 1 bit)")
      # "Stop bits"
      n131 = call-poly "VISA Configure Serial Port"("VISA resource name"=w380, "timeout (10sec)"=u32 10000, "baud rate (9600)"=u32 9600, "data bits (8)"=u16 8, "parity (0:none)"=enum16{"None", "Odd", "Even", "Mark", "Space"}."None", "stop bits (10: 1 bit)"=w377, "flow control (0:none)"=w378) -> ("VISA resource name out"=w373:refnum<visa-resource-name>, "error out"=w372:errorcluster)  [unwired: 7 in]
      "X COM PORT" <- w380
    }
    frame #1 {
      n132 = VISA Flush I/O Buffer(VISA resource name=w382) -> (VISA resource name out=w381:refnum<visa-resource-name>)  [unwired: 2 in, 1 out]
      n133 = call "mDrive Send Command.vi"("error in (no error)"=w384, "Extra"="EM 2", "Command"=T1."Send String", "VISA resource name"=w381) -> ("error out"=w383:errorcluster, "VISA resource name out"=w385:refnum<visa-resource-name>)  [unwired: 3 in, 1 out]
    }
    frame #2 {
      n134 = Number To Decimal String(number=1000000) -> (decimal integer string=w393:string)  [unwired: 1 in]
      n135 = call "mDrive Send Command.vi"("error in (no error)"=w390, "Extra"=w393, "Command"=T1."Accel Rate", "VISA resource name"=w389) -> ("error out"=w391:errorcluster, "VISA resource name out"=w397:refnum<visa-resource-name>)  [unwired: 3 in, 1 out]
      n136 = call "mDrive Send Command.vi"("error in (no error)"=w391, "Extra"=w393, "Command"=T1."Decel Rate", "VISA resource name"=w397) -> ("error out"=w392:errorcluster, "VISA resource name out"=w388:refnum<visa-resource-name>)  [unwired: 3 in, 1 out]
    }
    frame #3 {
      # "Run Current %"
      n137 = property on="X Run Current %" class="DigNum (strict)"() -> ("Value"=w399:i32)  [unwired: 2 in, 2 out]
      n138 = Number To Decimal String(number=w399) -> (decimal integer string=w400:string)  [unwired: 1 in]
      n139 = call "mDrive Send Command.vi"("error in (no error)"=w404, "Extra"=w400, "Command"=T1."Run Current", "VISA resource name"=w402) -> ("error out"=w403:errorcluster, "VISA resource name out"=w401:refnum<visa-resource-name>)  [unwired: 3 in, 1 out]
    }
    frame #4 {
      # "Holding Current %"
      n140 = property on="X Holding Current %" class="DigNum (strict)"() -> ("Value"=w406:i32)  [unwired: 2 in, 2 out]
      n141 = Number To Decimal String(number=w406) -> (decimal integer string=w407:string)  [unwired: 1 in]
      n142 = call "mDrive Send Command.vi"("error in (no error)"=w408, "Extra"=w407, "Command"=T1."Holding Current", "VISA resource name"=w411) -> ("error out"=w409:errorcluster, "VISA resource name out"=w410:refnum<visa-resource-name>)  [unwired: 3 in, 1 out]
    }
    frame #5 {
      # "Velocity Max"
      n143 = property on="X Velocity SP step/sec" class="DigNum (strict)"() -> ("Value"=w418:i32)  [unwired: 2 in, 2 out]
      n144 = Number To Decimal String(number=w418) -> (decimal integer string=w417:string)  [unwired: 1 in]
      n145 = call "mDrive Send Command.vi"("error in (no error)"=w419, "Extra"=w417, "Command"=T1."Max Velocity", "VISA resource name"=w420) -> ("error out"=w415:errorcluster, "VISA resource name out"=w425:refnum<visa-resource-name>)  [unwired: 3 in, 1 out]
      n146 = call "mDrive Send Command.vi"("error in (no error)"=w415, "Extra"="VM", "Command"=T1."Print Parameter", "VISA resource name"=w425) -> ("error out"=w422:errorcluster, "read buffer"=w423:string, "VISA resource name out"=w421:refnum<visa-resource-name>)  [unwired: 3 in]
      n147 = Decimal String To Number(string=w423, offset=0) -> (number=w416:i32)  [unwired: 1 in, 1 out]
      n148 = property on="X velocity PV step/sec" class="DigNum (strict)"("Val(Sgnl)"=w416) -> ()  [unwired: 2 in, 2 out]
    }
    frame #6 {
      # "PRINT POSITION"
      n149 = call "mDrive Send Command.vi"("error in (no error)"=w431, "Extra"="P", "Command"=T1."Print Parameter", "VISA resource name"=w432) -> ("error out"=w433:errorcluster, "read buffer"=w430:string, "VISA resource name out"=w434:refnum<visa-resource-name>)  [unwired: 3 in]
      n150 = Decimal String To Number(string=w430, offset=0) -> (number=w428:i32)  [unwired: 1 in, 1 out]
    }
    frame #7 {
      w437 = -2304000 ("lower limit")
      w438 = 2304000 ("upper limit")
      n151 = property on="X Step SP" class="DigNum (strict)"("Val(Sgnl)"=w435) -> ()  [unwired: 2 in, 2 out]
      n152 = property on="X Step SP" class="DigNum (strict)"("Maximum"=w438) -> ()  [unwired: 2 in, 2 out]
      n153 = property on="X Step SP" class="DigNum (strict)"("Minimum"=w437) -> ()  [unwired: 2 in, 2 out]
      n154 = In Range and Coerce(upper limit=w438, x=w435, lower limit=w437) -> (In Range?=w436:bool)  [unwired: 1 out]
      n155 = property on="APX:X_LIM" class="Bool (strict)"("Val(Sgnl)"=w436) -> ()  [unwired: 2 in, 2 out]
      "X MINPOS" <- w437
      "X MAXPOS" <- w438
    }
  }
  n156 = call-poly <vilib>:"Read From Spreadsheet File.vi"("file path (dialog if empty)"=path "S:/SSE/IMS/POS.TXT") -> ("first row"=w20:i64[])  [unwired: 6 in, 4 out]
  n157 = call-poly <vilib>:"Read From Spreadsheet File.vi"("file path (dialog if empty)"=path "S:/SSE/IMS/PRESET.TXT") -> ("all rows"=w8:string[][])  [unwired: 6 in, 4 out]
  n158 = Array To Cluster(array=w20) -> (cluster=w19:T3)
  n159 = Transpose 2D Array(2D array=w8) -> (transposed array=w9:string[][])
  n160 = Unbundle(w19) -> ("first row[0]"=w17:i64, "first row[1]"=w16:i64, "first row[2]"=w15:i64, "first row[3]"=w14:i64)  [unwired: 5 out]
  n161 = Delete From Array(array=w9, index (row)=0) -> (deleted portion=w10:string[], array with subset deleted=w12:string[][])  [unwired: 2 in]
  n162 = property on="Reset X Motor Steps" class="DigNum (strict)"("Val(Sgnl)"=w17) -> ()  [unwired: 2 in, 2 out]
  n163 = property on="Reset Y Motor Steps" class="DigNum (strict)"("Val(Sgnl)"=w16) -> ()  [unwired: 2 in, 2 out]
  n164 = property on="Reset Z Motor Steps" class="DigNum (strict)"("Val(Sgnl)"=w15) -> ()  [unwired: 2 in, 2 out]
  n165 = property on="Reset R Motor Steps" class="DigNum (strict)"("Val(Sgnl)"=w14) -> ()  [unwired: 2 in, 2 out]
  n166 = Transpose 2D Array(2D array=w12) -> (transposed array=w13:string[][])
  n167 = property on="Preset positions" class="Ring (strict)"("Strings []"=w10) -> ()  [unwired: 2 in, 2 out]
  n168 = Decimal String To Number(string=w13) -> (number=w11:i32[][])  [unwired: 2 in, 1 out]
  n169 = Initialize Array(w2, w2, 4 ("dimension size")) -> (w5:i32[][])
  n170 = Build Array (concatenate)(w5, w11) -> (→"Presets":i32[][])
  n171 = while {
    tunnel: w104 -> [w459]
    tunnel: w103 -> [w462]
    tunnel: [w463] -> w27
    tunnel: [w461] -> w28
    tunnel: w90 -> [w458]
    tunnel: w89 -> [w457]
    tunnel: [w456] -> w88
    tunnel: [w455] -> w87
    tunnel: w62 -> [w454]
    tunnel: w61 -> [w453]
    tunnel: [w452] -> w30
    tunnel: [w451] -> w29
    tunnel: w60 -> [w450]
    tunnel: w59 -> [w449]
    tunnel: [w448] -> w26
    tunnel: [w447] -> w25
    stop <- "stop" stop-if-true
    n172 = flat-sequence {
      frame #0 {
        n173 = call "DAQ Assistant"("number of samples"=100) -> ("data"=w469:dynamicdata)  [unwired: 16 in, 2 out]
        n174 = call "Convert from Dynamic Data"("Dynamic Data Type"=w469) -> ("Array"=w468:dbl[])  [unwired: 3 in]
        n175 = Add Array Elements(numeric array=w468) -> (sum=w467:dbl)
        n176 = Absolute Value(x=w467) -> (abs(x)=w464:dbl)
        "sum" <- w464
        n177 = Less?(x=w464, y=1.0) -> (x < y?=→"NC":bool)
      }
    }
    n178 = event shown="[0] Timeout" {
      selector: _ -> [_ _ _ _ _ _ _ _ _]
      dyn-events: _ -> [_ _ _ _ _ _ _ _ _]
      timeout: 100 -> [_ _ _ _ _ _ _ _ _]
      tunnel: w462 -> [w558 _ _ w1217 _ _ _ w1504 w1540]
      tunnel: [w557 _ _ w1223 _ _ _ w1502 w1538] -> w463
      tunnel: w459 -> [w502 _ _ w1218 _ _ _ w1505 w1541]
      tunnel: [w556 _ _ w1224 _ _ _ w1503 w1539] -> w461
      tunnel: w458 -> [w501 _ _ _ _ _ w1424 w1499 w1537]
      tunnel: w457 -> [w533 _ _ _ _ _ w1423 w1498 w1536]
      tunnel: [w532 _ _ _ _ _ w1422 w1501 w1535] -> w456
      tunnel: [w531 _ _ _ _ _ w1421 w1500 w1534] -> w455
      tunnel: w454 -> [w497 _ _ _ w1286 _ _ w1497 w1533]
      tunnel: w453 -> [w494 _ _ _ w1285 _ _ w1496 w1532]
      tunnel: [w508 _ _ _ w1283 _ _ w1495 w1529] -> w452
      tunnel: [w507 _ _ _ w1284 _ _ w1494 w1528] -> w451
      tunnel: w450 -> [w506 _ _ _ _ w1355 _ w1493 w1531]
      tunnel: w449 -> [w505 _ _ _ _ w1354 _ w1492 w1530]
      tunnel: [w504 _ _ _ _ w1352 _ w1491 w1527] -> w448
      tunnel: [w503 _ _ _ _ w1353 _ w1490 w1526] -> w447
      event Timeout {
        n179 = event-data() -> ()  [unwired: 1 in, 2 out]
        n180 = flat-sequence {
          tunnel: [w883] -> w544
          tunnel: [w861] -> w543
          tunnel: [w872] -> w542
          tunnel: [w852] -> w541
          tunnel: w501 -> [w851]
          tunnel: w533 -> [w850]
          tunnel: w544 -> [w894]
          tunnel: [w894] -> w540
          tunnel: w543 -> [w893]
          tunnel: [w893] -> w539
          tunnel: w542 -> [w892]
          tunnel: [w892] -> w538
          tunnel: w541 -> [w891]
          tunnel: [w891] -> w537
          tunnel: w540 -> [w897]
          tunnel: [w898] -> w536
          tunnel: w539 -> [w900]
          tunnel: [w899] -> w535
          tunnel: w538 -> [w896]
          tunnel: [w895] -> w534
          tunnel: w537 -> [w895]
          tunnel: w536 -> [w910]
          tunnel: w535 -> [w911]
          tunnel: w534 -> [w912]
          tunnel: [w909] -> w531
          tunnel: [w908] -> w532
          frame #0 {
            w856 = 0.1 ("Delay Time (s)")
            n181 = property on="X offset mm" class="DigNum (strict)"() -> ("Value"=w866:dbl)  [unwired: 2 in, 2 out]
            n182 = property on="X Step SP" class="DigNum (strict)"() -> ("Maximum"=w874:dbl)  [unwired: 2 in, 2 out]
            n183 = property on="X Step SP" class="DigNum (strict)"() -> ("Minimum"=w876:dbl)  [unwired: 2 in, 2 out]
            n184 = property on="X steps/rev" class="DigNum (strict)"() -> ("Value"=w870:u32)  [unwired: 2 in, 2 out]
            n185 = To Long Integer(number=w874) -> (32bit integer=w873:i32)
            n186 = To Long Integer(number=w876) -> (32bit integer=w875:i32)
            n187 = call "mDrive Send Command.vi"("error in (no error)"=w850, "Extra"="P", "Command"=T1."Print Parameter", "VISA resource name"=w851) -> ("error out"=w878:errorcluster, "read buffer"=w882:string, "VISA resource name out"=w880:refnum<visa-resource-name>)  [unwired: 3 in]
            n188 = call "Time Delay12"("error in (no error)"=w878, "Delay Time (s)"=w856) -> ("error out"=w877:errorcluster)  [unwired: 9 in]
            n189 = Decimal String To Number(string=w882, offset=0) -> (number=w863:i32)  [unwired: 1 in, 1 out]
            n190 = To Double Precision Float(number=w870) -> (double precision float=w871:dbl)
            n191 = To Long Integer(number=w863) -> (32bit integer=w864:i32)
            n192 = disable-structure shown="Disabled" {
              disable-tunnel: [w890 _] -> w883
              disable-tunnel: w880 -> [w889 _]
              disable-tunnel: [w888 _] -> w879
              disable-tunnel: w877 -> [w887 _]
              disable-tunnel: T1."Print Parameter" ("Command") -> [w886 _]
              disable-tunnel: "MV" ("Extra") -> [w885 _]
              disable-tunnel: [w884 _] -> w849
              frame Disabled {
                n193 = call "mDrive Send Command.vi"("error in (no error)"=w887, "Extra"=w885, "Command"=w886, "VISA resource name"=w889) -> ("error out"=w888:errorcluster, "read buffer"=w884:string, "VISA resource name out"=w890:refnum<visa-resource-name>)  [unwired: 3 in]
              }
              frame Enabled {
              }
            }
            n194 = property on="X Step PV" class="DigNum (strict)"("Val(Sgnl)"=w864) -> ()  [unwired: 2 in, 2 out]
            n195 = call "Time Delay11"("error in (no error)"=w879, "Delay Time (s)"=w856) -> ("error out"=w861:errorcluster)  [unwired: 9 in]
            n196 = In Range and Coerce(upper limit=w873, x=w864, lower limit=w875) -> (In Range?=w872:bool)  [unwired: 1 out]
            n197 = To Double Precision Float(number=w864) -> (double precision float=w865:dbl)
            n198 = Decimal String To Number(string=w849, offset=0 ("offset (0)")) -> (number=w855:i32)  [unwired: 1 in, 1 out]
            n199 = Not Equal?(x=w849, y="") -> (x != y?=w847:bool)
            n200 = property on="APX:X_LIM" class="Bool (strict)"("Val(Sgnl)"=w872) -> ()  [unwired: 2 in, 2 out]
            n201 = property on="APX:MX_RDY" class="Bool (strict)"("Val(Sgnl)"=w847) -> ()  [unwired: 2 in, 2 out]
            n202 = Divide(x=w865, y=w871) -> (x/y=w869:dbl)
            n203 = Number To Boolean Array(number=w855) -> (Boolean array=w854:bool[])
            n204 = property on="X mm/rev" class="DigNum (strict)"() -> ("Value"=w868:dbl)  [unwired: 2 in, 2 out]
            n205 = Index Array(array=w854, index=0) -> (element=w852:bool)
            n206 = property on="APX:MX_MVG" class="Bool (strict)"("Val(Sgnl)"=w852) -> ()  [unwired: 2 in, 2 out]
            n207 = Multiply(x=w869, y=w868) -> (x*y=w867:dbl)
            n208 = Add(x=w867, y=w866) -> (x+y=w846:dbl)
            n209 = property on="APX:MX_PV" class="DigNum (strict)"("Val(Sgnl)"=w846) -> ()  [unwired: 2 in, 2 out]
          }
          frame #1 {
          }
          frame #2 {
            n210 = case shown="False" w896 {
              tunnel: w897 -> [w903 w907]
              tunnel: [w904 w907] -> w898
              tunnel: [w905 w906] -> w899
              tunnel: w900 -> [w902 w906]
              frame False {
                n211 = call "mDrive Send Command.vi"("error in (no error)"=w902, "Command"=T1."Stop", "VISA resource name"=w903) -> ("error out"=w905:errorcluster, "VISA resource name out"=w904:refnum<visa-resource-name>)  [unwired: 4 in, 1 out]
              }
              frame True {
              }
            }
            "Boolean 2" <- w896
          }
          frame #3 {
            n212 = disable-structure shown="Disabled" {
              disable-tunnel: w912 -> [w918 _]
              disable-tunnel: w911 -> [w916 _]
              disable-tunnel: w910 -> [w915 _]
              disable-tunnel: [w914 _] -> w909
              disable-tunnel: [w913 _] -> w908
              frame Disabled {
                n213 = Implies(1:w918) -> (0:w917:bool, 2:w919:bool)
                n214 = case shown="False" w917 {
                  tunnel: w916 -> [w926 w979]
                  tunnel: w915 -> [w925 w980]
                  tunnel: [w924 w979] -> w914
                  tunnel: [w923 w980] -> w913
                  frame False {
                    # "Backlash"
                    n215 = flat-sequence {
                      tunnel: [w941] -> w938
                      tunnel: [w943] -> w937
                      tunnel: [w942] -> w936
                      tunnel: w926 -> [w940]
                      tunnel: w925 -> [w939]
                      tunnel: w938 -> [w951]
                      tunnel: [w951] -> w935
                      tunnel: w937 -> [w950]
                      tunnel: w936 -> [w949]
                      tunnel: [w948] -> w934
                      tunnel: [w947] -> w933
                      tunnel: [w946] -> w922
                      tunnel: w935 -> [w961]
                      tunnel: w934 -> [w960]
                      tunnel: w933 -> [w958]
                      tunnel: [w959] -> w932
                      tunnel: [w958] -> w931
                      tunnel: [w957] -> w928
                      tunnel: [w956] -> w927
                      tunnel: w922 -> [w956]
                      tunnel: w932 -> [w972]
                      tunnel: w931 -> [w965]
                      tunnel: [w972] -> w930
                      tunnel: [w971] -> w929
                      tunnel: w928 -> [w971]
                      tunnel: w927 -> [w967]
                      tunnel: [w966] -> w920
                      tunnel: w930 -> [w976]
                      tunnel: w929 -> [w975]
                      tunnel: [w974] -> w924
                      tunnel: [w973] -> w921
                      tunnel: w920 -> [w973]
                      tunnel: [w978] -> w923
                      tunnel: w921 -> [w978]
                      frame #0 {
                        n216 = property on="X Backlash steps/sec" class="DigNum (strict)"() -> ("Value"=w941:i32)  [unwired: 2 in, 2 out]
                        n217 = Number To Decimal String(number=w941) -> (decimal integer string=w944:string)  [unwired: 1 in]
                        n218 = call "mDrive Send Command.vi"("error in (no error)"=w940, "Extra"=w944, "Command"=T1."Max Velocity", "VISA resource name"=w939) -> ("error out"=w942:errorcluster, "VISA resource name out"=w943:refnum<visa-resource-name>)  [unwired: 3 in, 1 out]
                      }
                      frame #1 {
                        n219 = property on="X Backlash" class="DigNum (strict)"() -> ("Value"=w946:i32)  [unwired: 2 in, 2 out]
                        n220 = Number To Decimal String(number=w946) -> (decimal integer string=w952:string)  [unwired: 1 in]
                        n221 = call "mDrive Send Command.vi"("error in (no error)"=w949, "Extra"=w952, "Command"=T1."Move to Relative Position", "VISA resource name"=w950) -> ("error out"=w948:errorcluster, "VISA resource name out"=w947:refnum<visa-resource-name>)  [unwired: 3 in, 1 out]
                      }
                      frame #2 {
                        n222 = To Double Precision Float(number=w956) -> (double precision float=w954:dbl)
                        n223 = To Double Precision Float(number=w961) -> (double precision float=w963:dbl)
                        n224 = Absolute Value(x=w954) -> (abs(x)=w955:dbl)
                        n225 = Divide(x=w955, y=w963) -> (x/y=w964:dbl)
                        n226 = Add(x=w964, y=0.3) -> (x+y=w957:dbl)
                        n227 = call "Time Delay13"("error in (no error)"=w960, "Delay Time (s)"=w957) -> ("error out"=w959:errorcluster)  [unwired: 9 in]
                      }
                      frame #3 {
                        n228 = Negate(x=w967) -> (-x=w968:i32)
                        n229 = Number To Decimal String(number=w968) -> (decimal integer string=w969:string)  [unwired: 1 in]
                        n230 = call "mDrive Send Command.vi"("Extra"=w969, "Command"=T1."Move to Relative Position", "VISA resource name"=w965) -> ("VISA resource name out"=w966:refnum<visa-resource-name>)  [unwired: 4 in, 2 out]
                      }
                      frame #4 {
                        n231 = call "Time Delay14"("error in (no error)"=w976, "Delay Time (s)"=w975) -> ("error out"=w974:errorcluster)  [unwired: 9 in]
                      }
                      frame #5 {
                        w977 = FALSE ("Value (Signaling)")
                      }
                    }
                  }
                  frame True {
                  }
                }
              }
              frame Enabled {
              }
            }
          }
        }
        n232 = flat-sequence {
          tunnel: w558 -> [w1013]
          tunnel: w502 -> [w1012]
          tunnel: [w1018] -> w555
          tunnel: [w994] -> w553
          tunnel: [w1005] -> w551
          tunnel: [w985] -> w549
          tunnel: w555 -> [w1029]
          tunnel: [w1029] -> w554
          tunnel: w553 -> [w1028]
          tunnel: [w1028] -> w552
          tunnel: w551 -> [w1027]
          tunnel: [w1027] -> w550
          tunnel: w549 -> [w1026]
          tunnel: [w1026] -> w545
          tunnel: w554 -> [w1032]
          tunnel: [w1033] -> w548
          tunnel: w552 -> [w1035]
          tunnel: [w1034] -> w547
          tunnel: w550 -> [w1031]
          tunnel: [w1030] -> w546
          tunnel: w545 -> [w1030]
          tunnel: w548 -> [w1045]
          tunnel: w547 -> [w1046]
          tunnel: w546 -> [w1047]
          tunnel: [w1044] -> w557
          tunnel: [w1043] -> w556
          frame #0 {
            w989 = 0.1 ("Delay Time (s)")
            n233 = property on="Y offset mm" class="DigNum (strict)"() -> ("Value"=w999:dbl)  [unwired: 2 in, 2 out]
            n234 = property on="Y steps/rev" class="DigNum (strict)"() -> ("Value"=w1003:u32)  [unwired: 2 in, 2 out]
            n235 = property on="Y Step SP" class="DigNum (strict)"() -> ("Maximum"=w1007:dbl)  [unwired: 2 in, 2 out]
            n236 = property on="Y Step SP" class="DigNum (strict)"() -> ("Minimum"=w1009:dbl)  [unwired: 2 in, 2 out]
            n237 = To Long Integer(number=w1007) -> (32bit integer=w1006:i32)
            n238 = To Long Integer(number=w1009) -> (32bit integer=w1008:i32)
            n239 = call "mDrive Send Command.vi"("error in (no error)"=w1013, "Extra"="P", "Command"=T1."Print Parameter", "VISA resource name"=w1012) -> ("error out"=w1011:errorcluster, "read buffer"=w1017:string, "VISA resource name out"=w1015:refnum<visa-resource-name>)  [unwired: 3 in]
            "read buffer" <- w1017
            n240 = call "Time Delay4"("error in (no error)"=w1011, "Delay Time (s)"=w989) -> ("error out"=w1010:errorcluster)  [unwired: 9 in]
            n241 = Decimal String To Number(string=w1017, offset=0) -> (number=w996:i32)  [unwired: 1 in, 1 out]
            n242 = To Double Precision Float(number=w1003) -> (double precision float=w1004:dbl)
            n243 = To Long Integer(number=w996) -> (32bit integer=w997:i32)
            n244 = disable-structure shown="Disabled" {
              disable-tunnel: [w1025 _] -> w1018
              disable-tunnel: w1015 -> [w1024 _]
              disable-tunnel: [w1023 _] -> w1014
              disable-tunnel: w1010 -> [w1022 _]
              disable-tunnel: T1."Print Parameter" ("Command") -> [w1021 _]
              disable-tunnel: "MV" ("Extra") -> [w1020 _]
              disable-tunnel: [w1019 _] -> w982
              frame Disabled {
                n245 = call "mDrive Send Command.vi"("error in (no error)"=w1022, "Extra"=w1020, "Command"=w1021, "VISA resource name"=w1024) -> ("error out"=w1023:errorcluster, "read buffer"=w1019:string, "VISA resource name out"=w1025:refnum<visa-resource-name>)  [unwired: 3 in]
              }
              frame Enabled {
              }
            }
            n246 = property on="Y Step PV" class="DigNum (strict)"("Val(Sgnl)"=w997) -> ()  [unwired: 2 in, 2 out]
            n247 = call "Time Delay3"("error in (no error)"=w1014, "Delay Time (s)"=w989) -> ("error out"=w994:errorcluster)  [unwired: 9 in]
            n248 = In Range and Coerce(upper limit=w1006, x=w997, lower limit=w1008) -> (In Range?=w1005:bool)  [unwired: 1 out]
            n249 = To Double Precision Float(number=w997) -> (double precision float=w998:dbl)
            n250 = Decimal String To Number(string=w982, offset=0 ("offset (0)")) -> (number=w988:i32)  [unwired: 1 in, 1 out]
            n251 = Not Equal?(x=w982, y="") -> (x != y?=w983:bool)
            n252 = property on="APX:Y_LIM" class="Bool (strict)"("Val(Sgnl)"=w1005) -> ()  [unwired: 2 in, 2 out]
            n253 = property on="APX:MY_RDY" class="Bool (strict)"("Val(Sgnl)"=w983) -> ()  [unwired: 2 in, 2 out]
            n254 = Divide(x=w998, y=w1004) -> (x/y=w1002:dbl)
            n255 = Number To Boolean Array(number=w988) -> (Boolean array=w987:bool[])
            n256 = property on="Y mm/rev" class="DigNum (strict)"() -> ("Value"=w1001:dbl)  [unwired: 2 in, 2 out]
            n257 = Index Array(array=w987, index=0) -> (element=w985:bool)
            n258 = property on="APX:MY_MVG" class="Bool (strict)"("Val(Sgnl)"=w985) -> ()  [unwired: 2 in, 2 out]
            n259 = Multiply(x=w1002, y=w1001) -> (x*y=w1000:dbl)
            n260 = Add(x=w1000, y=w999) -> (x+y=w981:dbl)
            n261 = property on="APX:MY_PV" class="DigNum (strict)"("Val(Sgnl)"=w981) -> ()  [unwired: 2 in, 2 out]
          }
          frame #1 {
          }
          frame #2 {
            n262 = case shown="False" w1031 {
              tunnel: w1032 -> [w1038 w1042]
              tunnel: [w1039 w1042] -> w1033
              tunnel: [w1040 w1041] -> w1034
              tunnel: w1035 -> [w1037 w1041]
              frame False {
                n263 = call "mDrive Send Command.vi"("error in (no error)"=w1037, "Command"=T1."Stop", "VISA resource name"=w1038) -> ("error out"=w1040:errorcluster, "VISA resource name out"=w1039:refnum<visa-resource-name>)  [unwired: 4 in, 1 out]
              }
              frame True {
              }
            }
            "Boolean" <- w1031
          }
          frame #3 {
            n264 = disable-structure shown="Disabled" {
              disable-tunnel: w1047 -> [w1053 _]
              disable-tunnel: w1046 -> [w1051 _]
              disable-tunnel: w1045 -> [w1050 _]
              disable-tunnel: [w1049 _] -> w1044
              disable-tunnel: [w1048 _] -> w1043
              frame Disabled {
                n265 = Implies(1:w1053) -> (0:w1052:bool, 2:w1054:bool)
                n266 = case shown="False" w1052 {
                  tunnel: w1051 -> [w1061 w1114]
                  tunnel: w1050 -> [w1060 w1115]
                  tunnel: [w1059 w1114] -> w1049
                  tunnel: [w1058 w1115] -> w1048
                  frame False {
                    # "Backlash"
                    n267 = flat-sequence {
                      tunnel: [w1076] -> w1073
                      tunnel: [w1078] -> w1072
                      tunnel: [w1077] -> w1071
                      tunnel: w1061 -> [w1075]
                      tunnel: w1060 -> [w1074]
                      tunnel: w1073 -> [w1086]
                      tunnel: [w1086] -> w1070
                      tunnel: w1072 -> [w1085]
                      tunnel: w1071 -> [w1084]
                      tunnel: [w1083] -> w1069
                      tunnel: [w1082] -> w1068
                      tunnel: [w1081] -> w1057
                      tunnel: w1070 -> [w1096]
                      tunnel: w1069 -> [w1095]
                      tunnel: w1068 -> [w1093]
                      tunnel: [w1094] -> w1067
                      tunnel: [w1093] -> w1066
                      tunnel: [w1092] -> w1063
                      tunnel: [w1091] -> w1062
                      tunnel: w1057 -> [w1091]
                      tunnel: w1067 -> [w1107]
                      tunnel: w1066 -> [w1100]
                      tunnel: [w1107] -> w1065
                      tunnel: [w1106] -> w1064
                      tunnel: w1063 -> [w1106]
                      tunnel: w1062 -> [w1102]
                      tunnel: [w1101] -> w1055
                      tunnel: w1065 -> [w1111]
                      tunnel: w1064 -> [w1110]
                      tunnel: [w1109] -> w1059
                      tunnel: [w1108] -> w1056
                      tunnel: w1055 -> [w1108]
                      tunnel: [w1113] -> w1058
                      tunnel: w1056 -> [w1113]
                      frame #0 {
                        n268 = property on="Y Backlash steps/sec" class="DigNum (strict)"() -> ("Value"=w1076:i32)  [unwired: 2 in, 2 out]
                        n269 = Number To Decimal String(number=w1076) -> (decimal integer string=w1079:string)  [unwired: 1 in]
                        n270 = call "mDrive Send Command.vi"("error in (no error)"=w1075, "Extra"=w1079, "Command"=T1."Max Velocity", "VISA resource name"=w1074) -> ("error out"=w1077:errorcluster, "VISA resource name out"=w1078:refnum<visa-resource-name>)  [unwired: 3 in, 1 out]
                      }
                      frame #1 {
                        n271 = property on="Y Backlash" class="DigNum (strict)"() -> ("Value"=w1081:i32)  [unwired: 2 in, 2 out]
                        n272 = Number To Decimal String(number=w1081) -> (decimal integer string=w1087:string)  [unwired: 1 in]
                        n273 = call "mDrive Send Command.vi"("error in (no error)"=w1084, "Extra"=w1087, "Command"=T1."Move to Relative Position", "VISA resource name"=w1085) -> ("error out"=w1083:errorcluster, "VISA resource name out"=w1082:refnum<visa-resource-name>)  [unwired: 3 in, 1 out]
                      }
                      frame #2 {
                        n274 = To Double Precision Float(number=w1091) -> (double precision float=w1089:dbl)
                        n275 = To Double Precision Float(number=w1096) -> (double precision float=w1098:dbl)
                        n276 = Absolute Value(x=w1089) -> (abs(x)=w1090:dbl)
                        n277 = Divide(x=w1090, y=w1098) -> (x/y=w1099:dbl)
                        n278 = Add(x=w1099, y=0.3) -> (x+y=w1092:dbl)
                        n279 = call "Time Delay8"("error in (no error)"=w1095, "Delay Time (s)"=w1092) -> ("error out"=w1094:errorcluster)  [unwired: 9 in]
                      }
                      frame #3 {
                        n280 = Negate(x=w1102) -> (-x=w1103:i32)
                        n281 = Number To Decimal String(number=w1103) -> (decimal integer string=w1104:string)  [unwired: 1 in]
                        n282 = call "mDrive Send Command.vi"("Extra"=w1104, "Command"=T1."Move to Relative Position", "VISA resource name"=w1100) -> ("VISA resource name out"=w1101:refnum<visa-resource-name>)  [unwired: 4 in, 2 out]
                      }
                      frame #4 {
                        n283 = call "Time Delay2"("error in (no error)"=w1111, "Delay Time (s)"=w1110) -> ("error out"=w1109:errorcluster)  [unwired: 9 in]
                      }
                      frame #5 {
                        w1112 = FALSE ("Value (Signaling)")
                      }
                    }
                  }
                  frame True {
                  }
                }
              }
              frame Enabled {
              }
            }
          }
        }
        n284 = flat-sequence {
          tunnel: [w748] -> w530
          tunnel: [w727] -> w529
          tunnel: [w738] -> w528
          tunnel: [w718] -> w527
          tunnel: w496 -> [w717]
          tunnel: w495 -> [w716]
          tunnel: w530 -> [w759]
          tunnel: [w759] -> w526
          tunnel: w529 -> [w758]
          tunnel: [w758] -> w525
          tunnel: w528 -> [w757]
          tunnel: [w757] -> w524
          tunnel: w527 -> [w756]
          tunnel: [w756] -> w523
          tunnel: w526 -> [w762]
          tunnel: [w763] -> w522
          tunnel: w525 -> [w765]
          tunnel: [w764] -> w521
          tunnel: w524 -> [w761]
          tunnel: [w760] -> w520
          tunnel: w523 -> [w760]
          tunnel: w522 -> [w775]
          tunnel: w521 -> [w776]
          tunnel: w520 -> [w777]
          tunnel: [w774] -> w507
          tunnel: [w773] -> w508
          frame #0 {
            w722 = 0.1 ("Delay Time (s)")
            n285 = property on="Z Step SP" class="DigNum (strict)" props=["Maximum"]() -> ()  [unwired: 2 in, 3 out]
            n286 = property on="Z offset mm" class="DigNum (strict)"() -> ("Value"=w732:dbl)  [unwired: 2 in, 2 out]
            n287 = property on="Z steps/rev" class="DigNum (strict)"() -> ("Value"=w736:u32)  [unwired: 2 in, 2 out]
            n288 = property on="Z Step SP" class="DigNum (strict)"() -> ("Minimum"=w741:dbl)  [unwired: 2 in, 2 out]
            n289 = property on="Z max step" class="DigNum (strict)"() -> ("Value"=w712:i32)  [unwired: 2 in, 2 out]
            n290 = To Long Integer(number=w712) -> (32bit integer=w739:i32)
            n291 = To Long Integer(number=w741) -> (32bit integer=w740:i32)
            n292 = call "mDrive Send Command.vi"("error in (no error)"=w716, "Extra"="P", "Command"=T1."Print Parameter", "VISA resource name"=w717) -> ("error out"=w743:errorcluster, "read buffer"=w747:string, "VISA resource name out"=w745:refnum<visa-resource-name>)  [unwired: 3 in]
            n293 = call "Time Delay17"("error in (no error)"=w743, "Delay Time (s)"=w722) -> ("error out"=w742:errorcluster)  [unwired: 9 in]
            n294 = Decimal String To Number(string=w747, offset=0) -> (number=w729:i32)  [unwired: 1 in, 1 out]
            n295 = To Double Precision Float(number=w736) -> (double precision float=w737:dbl)
            n296 = To Long Integer(number=w729) -> (32bit integer=w730:i32)
            n297 = property on="Z Step PV" class="DigNum (strict)"("Val(Sgnl)"=w730) -> ()  [unwired: 2 in, 2 out]
            n298 = disable-structure shown="Disabled" {
              disable-tunnel: [w755 _] -> w748
              disable-tunnel: w745 -> [w754 _]
              disable-tunnel: [w753 _] -> w744
              disable-tunnel: w742 -> [w752 _]
              disable-tunnel: T1."Print Parameter" ("Command") -> [w751 _]
              disable-tunnel: "MV" ("Extra") -> [w750 _]
              disable-tunnel: [w749 _] -> w713
              frame Disabled {
                n299 = call "mDrive Send Command.vi"("error in (no error)"=w752, "Extra"=w750, "Command"=w751, "VISA resource name"=w754) -> ("error out"=w753:errorcluster, "read buffer"=w749:string, "VISA resource name out"=w755:refnum<visa-resource-name>)  [unwired: 3 in]
              }
              frame Enabled {
              }
            }
            n300 = call "Time Delay16"("error in (no error)"=w744, "Delay Time (s)"=w722) -> ("error out"=w727:errorcluster)  [unwired: 9 in]
            n301 = In Range and Coerce(upper limit=w739, x=w730, lower limit=w740) -> (In Range?=w738:bool)  [unwired: 1 out]
            n302 = To Double Precision Float(number=w730) -> (double precision float=w731:dbl)
            n303 = Decimal String To Number(string=w713, offset=0 ("offset (0)")) -> (number=w721:i32)  [unwired: 1 in, 1 out]
            n304 = Not Equal?(x=w713, y="") -> (x != y?=w714:bool)
            n305 = property on="APX:MZ_LIM" class="Bool (strict)"("Val(Sgnl)"=w738) -> ()  [unwired: 2 in, 2 out]
            n306 = property on="APX:MZ_RDY" class="Bool (strict)"("Val(Sgnl)"=w714) -> ()  [unwired: 2 in, 2 out]
            n307 = Divide(x=w731, y=w737) -> (x/y=w735:dbl)
            n308 = Number To Boolean Array(number=w721) -> (Boolean array=w720:bool[])
            n309 = property on="Z mm/rev" class="DigNum (strict)"() -> ("Value"=w734:dbl)  [unwired: 2 in, 2 out]
            n310 = Index Array(array=w720, index=0) -> (element=w718:bool)
            n311 = property on="APX:MZ_MVG" class="Bool (strict)"("Val(Sgnl)"=w718) -> ()  [unwired: 2 in, 2 out]
            n312 = Multiply(x=w735, y=w734) -> (x*y=w733:dbl)
            n313 = Add(x=w733, y=w732) -> (x+y=w711:dbl)
            n314 = property on="APX:MZ_PV" class="DigNum (strict)"("Val(Sgnl)"=w711) -> ()  [unwired: 2 in, 2 out]
          }
          frame #1 {
          }
          frame #2 {
            n315 = case shown="True" w761 {
              tunnel: w762 -> [w768 w772]
              tunnel: [w769 w772] -> w763
              tunnel: [w770 w771] -> w764
              tunnel: w765 -> [w767 w771]
              frame False {
                n316 = call "mDrive Send Command.vi"("error in (no error)"=w767, "Command"=T1."Stop", "VISA resource name"=w768) -> ("error out"=w770:errorcluster, "VISA resource name out"=w769:refnum<visa-resource-name>)  [unwired: 4 in, 1 out]
              }
              frame True {
              }
            }
            "Boolean 3" <- w761
          }
          frame #3 {
            n317 = disable-structure shown="Disabled" {
              disable-tunnel: w777 -> [w783 _]
              disable-tunnel: w776 -> [w781 _]
              disable-tunnel: w775 -> [w780 _]
              disable-tunnel: [w779 _] -> w774
              disable-tunnel: [w778 _] -> w773
              frame Disabled {
                n318 = Implies(1:w783) -> (0:w782:bool, 2:w784:bool)
                n319 = case shown="False" w782 {
                  tunnel: w781 -> [w791 w844]
                  tunnel: w780 -> [w790 w845]
                  tunnel: [w789 w844] -> w779
                  tunnel: [w788 w845] -> w778
                  frame False {
                    # "Backlash"
                    n320 = flat-sequence {
                      tunnel: [w806] -> w803
                      tunnel: [w808] -> w802
                      tunnel: [w807] -> w801
                      tunnel: w791 -> [w805]
                      tunnel: w790 -> [w804]
                      tunnel: w803 -> [w816]
                      tunnel: [w816] -> w800
                      tunnel: w802 -> [w815]
                      tunnel: w801 -> [w814]
                      tunnel: [w813] -> w799
                      tunnel: [w812] -> w798
                      tunnel: [w811] -> w787
                      tunnel: w800 -> [w826]
                      tunnel: w799 -> [w825]
                      tunnel: w798 -> [w823]
                      tunnel: [w824] -> w797
                      tunnel: [w823] -> w796
                      tunnel: [w822] -> w793
                      tunnel: [w821] -> w792
                      tunnel: w787 -> [w821]
                      tunnel: w797 -> [w837]
                      tunnel: w796 -> [w830]
                      tunnel: [w837] -> w795
                      tunnel: [w836] -> w794
                      tunnel: w793 -> [w836]
                      tunnel: w792 -> [w832]
                      tunnel: [w831] -> w785
                      tunnel: w795 -> [w841]
                      tunnel: w794 -> [w840]
                      tunnel: [w839] -> w789
                      tunnel: [w838] -> w786
                      tunnel: w785 -> [w838]
                      tunnel: [w843] -> w788
                      tunnel: w786 -> [w843]
                      frame #0 {
                        n321 = property on="Z Backlash steps/sec" class="DigNum (strict)"() -> ("Value"=w806:i32)  [unwired: 2 in, 2 out]
                        n322 = Number To Decimal String(number=w806) -> (decimal integer string=w809:string)  [unwired: 1 in]
                        n323 = call "mDrive Send Command.vi"("error in (no error)"=w805, "Extra"=w809, "Command"=T1."Max Velocity", "VISA resource name"=w804) -> ("error out"=w807:errorcluster, "VISA resource name out"=w808:refnum<visa-resource-name>)  [unwired: 3 in, 1 out]
                      }
                      frame #1 {
                        n324 = property on="Z Backlash" class="DigNum (strict)"() -> ("Value"=w811:i32)  [unwired: 2 in, 2 out]
                        n325 = Number To Decimal String(number=w811) -> (decimal integer string=w817:string)  [unwired: 1 in]
                        n326 = call "mDrive Send Command.vi"("error in (no error)"=w814, "Extra"=w817, "Command"=T1."Move to Relative Position", "VISA resource name"=w815) -> ("error out"=w813:errorcluster, "VISA resource name out"=w812:refnum<visa-resource-name>)  [unwired: 3 in, 1 out]
                      }
                      frame #2 {
                        n327 = To Double Precision Float(number=w821) -> (double precision float=w819:dbl)
                        n328 = To Double Precision Float(number=w826) -> (double precision float=w828:dbl)
                        n329 = Absolute Value(x=w819) -> (abs(x)=w820:dbl)
                        n330 = Divide(x=w820, y=w828) -> (x/y=w829:dbl)
                        n331 = Add(x=w829, y=0.5) -> (x+y=w822:dbl)
                        n332 = call "Time Delay18"("error in (no error)"=w825, "Delay Time (s)"=w822) -> ("error out"=w824:errorcluster)  [unwired: 9 in]
                      }
                      frame #3 {
                        n333 = Negate(x=w832) -> (-x=w833:i32)
                        n334 = Number To Decimal String(number=w833) -> (decimal integer string=w834:string)  [unwired: 1 in]
                        n335 = call "mDrive Send Command.vi"("Extra"=w834, "Command"=T1."Move to Relative Position", "VISA resource name"=w830) -> ("VISA resource name out"=w831:refnum<visa-resource-name>)  [unwired: 4 in, 2 out]
                      }
                      frame #4 {
                        n336 = call "Time Delay19"("error in (no error)"=w841, "Delay Time (s)"=w840) -> ("error out"=w839:errorcluster)  [unwired: 9 in]
                      }
                      frame #5 {
                        w842 = FALSE ("Value (Signaling)")
                      }
                    }
                  }
                  frame True {
                  }
                }
              }
              frame Enabled {
              }
            }
          }
        }
        n337 = flat-sequence {
          tunnel: [w613] -> w519
          tunnel: [w591] -> w518
          tunnel: [w602] -> w517
          tunnel: [w582] -> w516
          tunnel: w506 -> [w581]
          tunnel: w505 -> [w580]
          tunnel: w519 -> [w624]
          tunnel: [w624] -> w515
          tunnel: w518 -> [w623]
          tunnel: [w623] -> w514
          tunnel: w517 -> [w622]
          tunnel: [w622] -> w513
          tunnel: w516 -> [w621]
          tunnel: [w621] -> w512
          tunnel: w515 -> [w627]
          tunnel: [w628] -> w511
          tunnel: w514 -> [w630]
          tunnel: [w629] -> w510
          tunnel: w513 -> [w626]
          tunnel: [w625] -> w509
          tunnel: w512 -> [w625]
          tunnel: w511 -> [w640]
          tunnel: w510 -> [w641]
          tunnel: w509 -> [w642]
          tunnel: [w639] -> w503
          tunnel: [w638] -> w504
          frame #0 {
            w586 = 0.1 ("Delay Time (s)")
            n338 = property on="R offset deg" class="DigNum (strict)"() -> ("Value"=w596:dbl)  [unwired: 2 in, 2 out]
            n339 = property on="R steps/rev" class="DigNum (strict)"() -> ("Value"=w600:u32)  [unwired: 2 in, 2 out]
            n340 = property on="R Step SP" class="DigNum (strict)"() -> ("Maximum"=w604:dbl)  [unwired: 2 in, 2 out]
            n341 = property on="R Step SP" class="DigNum (strict)"() -> ("Minimum"=w606:dbl)  [unwired: 2 in, 2 out]
            n342 = To Long Integer(number=w604) -> (32bit integer=w603:i32)
            n343 = To Long Integer(number=w606) -> (32bit integer=w605:i32)
            n344 = call "mDrive Send Command.vi"("error in (no error)"=w580, "Extra"="P", "Command"=T1."Print Parameter", "VISA resource name"=w581) -> ("error out"=w608:errorcluster, "read buffer"=w612:string, "VISA resource name out"=w610:refnum<visa-resource-name>)  [unwired: 3 in]
            n345 = call "Time Delay21"("error in (no error)"=w608, "Delay Time (s)"=w586) -> ("error out"=w607:errorcluster)  [unwired: 9 in]
            n346 = Decimal String To Number(string=w612, offset=0) -> (number=w593:i32)  [unwired: 1 in, 1 out]
            n347 = To Double Precision Float(number=w600) -> (double precision float=w601:dbl)
            n348 = To Long Integer(number=w593) -> (32bit integer=w594:i32)
            n349 = disable-structure shown="Disabled" {
              disable-tunnel: [w620 _] -> w613
              disable-tunnel: w610 -> [w619 _]
              disable-tunnel: [w618 _] -> w609
              disable-tunnel: w607 -> [w617 _]
              disable-tunnel: T1."Print Parameter" ("Command") -> [w616 _]
              disable-tunnel: "MV" ("Extra") -> [w615 _]
              disable-tunnel: [w614 _] -> w577
              frame Disabled {
                n350 = call "mDrive Send Command.vi"("error in (no error)"=w617, "Extra"=w615, "Command"=w616, "VISA resource name"=w619) -> ("error out"=w618:errorcluster, "read buffer"=w614:string, "VISA resource name out"=w620:refnum<visa-resource-name>)  [unwired: 3 in]
              }
              frame Enabled {
              }
            }
            n351 = property on="R Step PV" class="DigNum (strict)"("Val(Sgnl)"=w594) -> ()  [unwired: 2 in, 2 out]
            n352 = call "Time Delay20"("error in (no error)"=w609, "Delay Time (s)"=w586) -> ("error out"=w591:errorcluster)  [unwired: 9 in]
            n353 = In Range and Coerce(upper limit=w603, x=w594, lower limit=w605) -> (In Range?=w602:bool)  [unwired: 1 out]
            n354 = To Double Precision Float(number=w594) -> (double precision float=w595:dbl)
            n355 = Decimal String To Number(string=w577, offset=0 ("offset (0)")) -> (number=w585:i32)  [unwired: 1 in, 1 out]
            n356 = Not Equal?(x=w577, y="") -> (x != y?=w578:bool)
            n357 = property on="APX:MR_LIM" class="Bool (strict)"("Val(Sgnl)"=w602) -> ()  [unwired: 2 in, 2 out]
            n358 = property on="APX:MR_RDY" class="Bool (strict)"("Val(Sgnl)"=w578) -> ()  [unwired: 2 in, 2 out]
            n359 = Divide(x=w595, y=w601) -> (x/y=w599:dbl)
            n360 = Number To Boolean Array(number=w585) -> (Boolean array=w584:bool[])
            n361 = property on="R deg/rev" class="DigNum (strict)"() -> ("Value"=w598:dbl)  [unwired: 2 in, 2 out]
            n362 = Index Array(array=w584, index=0) -> (element=w582:bool)
            n363 = property on="APX:MR_MVG" class="Bool (strict)"("Val(Sgnl)"=w582) -> ()  [unwired: 2 in, 2 out]
            n364 = Multiply(x=w599, y=w598) -> (x*y=w597:dbl)
            n365 = Add(x=w597, y=w596) -> (x+y=w576:dbl)
            n366 = property on="APZ:MR_PV" class="DigNum (strict)"("Val(Sgnl)"=w576) -> ()  [unwired: 2 in, 2 out]
          }
          frame #1 {
          }
          frame #2 {
            n367 = case shown="False" w626 {
              tunnel: w627 -> [w633 w637]
              tunnel: [w634 w637] -> w628
              tunnel: [w635 w636] -> w629
              tunnel: w630 -> [w632 w636]
              frame False {
                n368 = call "mDrive Send Command.vi"("error in (no error)"=w632, "Command"=T1."Stop", "VISA resource name"=w633) -> ("error out"=w635:errorcluster, "VISA resource name out"=w634:refnum<visa-resource-name>)  [unwired: 4 in, 1 out]
              }
              frame True {
              }
            }
          }
          frame #3 {
            n369 = disable-structure shown="Disabled" {
              disable-tunnel: w642 -> [w648 _]
              disable-tunnel: w641 -> [w646 _]
              disable-tunnel: w640 -> [w645 _]
              disable-tunnel: [w644 _] -> w639
              disable-tunnel: [w643 _] -> w638
              frame Disabled {
                n370 = Implies(1:w648) -> (0:w647:bool, 2:w649:bool)
                n371 = case shown="False" w647 {
                  tunnel: w646 -> [w656 w709]
                  tunnel: w645 -> [w655 w710]
                  tunnel: [w654 w709] -> w644
                  tunnel: [w653 w710] -> w643
                  frame False {
                    # "Backlash"
                    n372 = flat-sequence {
                      tunnel: [w671] -> w668
                      tunnel: [w673] -> w667
                      tunnel: [w672] -> w666
                      tunnel: w656 -> [w670]
                      tunnel: w655 -> [w669]
                      tunnel: w668 -> [w681]
                      tunnel: [w681] -> w665
                      tunnel: w667 -> [w680]
                      tunnel: w666 -> [w679]
                      tunnel: [w678] -> w664
                      tunnel: [w677] -> w663
                      tunnel: [w676] -> w652
                      tunnel: w665 -> [w691]
                      tunnel: w664 -> [w690]
                      tunnel: w663 -> [w688]
                      tunnel: [w689] -> w662
                      tunnel: [w688] -> w661
                      tunnel: [w687] -> w658
                      tunnel: [w686] -> w657
                      tunnel: w652 -> [w686]
                      tunnel: w662 -> [w702]
                      tunnel: w661 -> [w695]
                      tunnel: [w702] -> w660
                      tunnel: [w701] -> w659
                      tunnel: w658 -> [w701]
                      tunnel: w657 -> [w697]
                      tunnel: [w696] -> w650
                      tunnel: w660 -> [w706]
                      tunnel: w659 -> [w705]
                      tunnel: [w704] -> w654
                      tunnel: [w703] -> w651
                      tunnel: w650 -> [w703]
                      tunnel: [w708] -> w653
                      tunnel: w651 -> [w708]
                      frame #0 {
                        n373 = property on="R Backlash steps/sec" class="DigNum (strict)"() -> ("Value"=w671:i32)  [unwired: 2 in, 2 out]
                        n374 = Number To Decimal String(number=w671) -> (decimal integer string=w674:string)  [unwired: 1 in]
                        n375 = call "mDrive Send Command.vi"("error in (no error)"=w670, "Extra"=w674, "Command"=T1."Max Velocity", "VISA resource name"=w669) -> ("error out"=w672:errorcluster, "VISA resource name out"=w673:refnum<visa-resource-name>)  [unwired: 3 in, 1 out]
                      }
                      frame #1 {
                        n376 = property on="R Backlash" class="DigNum (strict)"() -> ("Value"=w676:i32)  [unwired: 2 in, 2 out]
                        n377 = Number To Decimal String(number=w676) -> (decimal integer string=w682:string)  [unwired: 1 in]
                        n378 = call "mDrive Send Command.vi"("error in (no error)"=w679, "Extra"=w682, "Command"=T1."Move to Relative Position", "VISA resource name"=w680) -> ("error out"=w678:errorcluster, "VISA resource name out"=w677:refnum<visa-resource-name>)  [unwired: 3 in, 1 out]
                      }
                      frame #2 {
                        n379 = To Double Precision Float(number=w686) -> (double precision float=w684:dbl)
                        n380 = To Double Precision Float(number=w691) -> (double precision float=w693:dbl)
                        n381 = Absolute Value(x=w684) -> (abs(x)=w685:dbl)
                        n382 = Divide(x=w685, y=w693) -> (x/y=w694:dbl)
                        n383 = Add(x=w694, y=0.3) -> (x+y=w687:dbl)
                        n384 = call "Time Delay22"("error in (no error)"=w690, "Delay Time (s)"=w687) -> ("error out"=w689:errorcluster)  [unwired: 9 in]
                      }
                      frame #3 {
                        n385 = Negate(x=w697) -> (-x=w698:i32)
                        n386 = Number To Decimal String(number=w698) -> (decimal integer string=w699:string)  [unwired: 1 in]
                        n387 = call "mDrive Send Command.vi"("Extra"=w699, "Command"=T1."Move to Relative Position", "VISA resource name"=w695) -> ("VISA resource name out"=w696:refnum<visa-resource-name>)  [unwired: 4 in, 2 out]
                      }
                      frame #4 {
                        n388 = call "Time Delay23"("error in (no error)"=w706, "Delay Time (s)"=w705) -> ("error out"=w704:errorcluster)  [unwired: 9 in]
                      }
                      frame #5 {
                        w707 = FALSE ("Value (Signaling)")
                      }
                    }
                  }
                  frame True {
                  }
                }
              }
              frame Enabled {
              }
            }
          }
        }
        n389 = property on="Open?" class="Bool (strict)"() -> ("Value"=w500:bool)  [unwired: 2 in, 2 out]
        n390 = disable-structure shown="Disabled" {
          frame Disabled {
            n391 = Divide() -> (x=w566:dbl, y=w567:dbl, x/y=w568:dbl)
            n392 = Inverse Tangent(1:w568) -> (0:w569:dbl)
            n393 = Divide(x=w569, y=6.283185307179586) -> (x/y=w570:dbl)
            n394 = Multiply(x=360.0, y=w570) -> (x*y=w573:dbl)
          }
          frame Enabled {
          }
        }
        n395 = case shown="False" w500 {
          tunnel: [w574 w575] -> w499
          frame False {
            n396 = property on="V5 position 15360000" class="DigNum (strict)"() -> ("Value"=w574:i32)  [unwired: 2 in, 2 out]
          }
          frame True {
            n397 = property on="Z Step SP" class="DigNum (strict)"() -> ("Maximum"=w575:dbl)  [unwired: 2 in, 2 out]
          }
        }
        "Z max step" <- w499
        n398 = property on="NC" class="Bool (strict)"() -> ("Value"=w498:bool)  [unwired: 2 in, 2 out]
        n399 = case shown="False" w498 {
          tunnel: w497 -> [w563 w565]
          tunnel: [w562 w565] -> w496
          tunnel: w494 -> [w560 w564]
          tunnel: [w559 w564] -> w495
          frame False {
            n400 = call "mDrive Send Command.vi"("error in (no error)"=w560, "Command"=T1."Stop", "VISA resource name"=w563) -> ("error out"=w559:errorcluster, "VISA resource name out"=w562:refnum<visa-resource-name>)  [unwired: 4 in, 1 out]
          }
          frame True {
          }
        }
      }
      event "Reset Y Position mm", "Reset X Position mm", "Reset Z Position mm", "Reset R Position deg": Value Change {
        n401 = event-data() -> ()  [unwired: 1 in, 5 out]
        n402 = property on="Y offset mm" class="DigNum (strict)"() -> ("Value"=w1143:dbl)  [unwired: 2 in, 2 out]
        n403 = property on="X offset mm" class="DigNum (strict)"() -> ("Value"=w1134:dbl)  [unwired: 2 in, 2 out]
        n404 = property on="R offset deg" class="DigNum (strict)"() -> ("Value"=w1116:dbl)  [unwired: 2 in, 2 out]
        n405 = property on="Y steps/rev" class="DigNum (strict)"() -> ("Value"=w1145:u32)  [unwired: 2 in, 2 out]
        n406 = property on="X steps/rev" class="DigNum (strict)"() -> ("Value"=w1136:u32)  [unwired: 2 in, 2 out]
        n407 = property on="R steps/rev" class="DigNum (strict)"() -> ("Value"=w1118:u32)  [unwired: 2 in, 2 out]
        n408 = property on="Z steps/rev" class="DigNum (strict)"() -> ("Value"=w1127:u32)  [unwired: 2 in, 2 out]
        n409 = property on="Reset Y Position mm" class="DigNum (strict)"() -> ("Value"=w1151:dbl)  [unwired: 2 in, 2 out]
        n410 = property on="Reset X Position mm" class="DigNum (strict)"() -> ("Value"=w1142:dbl)  [unwired: 2 in, 2 out]
        n411 = property on="Reset Z Position mm" class="DigNum (strict)"() -> ("Value"=w1133:dbl)  [unwired: 2 in, 2 out]
        n412 = property on="Reset R Position deg" class="DigNum (strict)"() -> ("Value"=w1124:dbl)  [unwired: 2 in, 2 out]
        n413 = property on="Z offset mm" class="DigNum (strict)"() -> ("Value"=w1125:dbl)  [unwired: 2 in, 2 out]
        n414 = Subtract(x=w1151, y=w1143) -> (x-y=w1150:dbl)
        n415 = Subtract(x=w1142, y=w1134) -> (x-y=w1141:dbl)
        n416 = Subtract(x=w1124, y=w1116) -> (x-y=w1123:dbl)
        n417 = Subtract(x=w1133, y=w1125) -> (x-y=w1132:dbl)
        n418 = To Double Precision Float(number=w1136) -> (double precision float=w1139:dbl)
        n419 = To Double Precision Float(number=w1127) -> (double precision float=w1130:dbl)
        n420 = property on="Y mm/rev" class="DigNum (strict)"() -> ("Value"=w1144:dbl)  [unwired: 2 in, 2 out]
        n421 = property on="X mm/rev" class="DigNum (strict)"() -> ("Value"=w1135:dbl)  [unwired: 2 in, 2 out]
        n422 = property on="Z mm/rev" class="DigNum (strict)"() -> ("Value"=w1126:dbl)  [unwired: 2 in, 2 out]
        n423 = property on="R deg/rev" class="DigNum (strict)"() -> ("Value"=w1117:dbl)  [unwired: 2 in, 2 out]
        n424 = Divide(x=w1150, y=w1144) -> (x/y=w1149:dbl)
        n425 = Divide(x=w1141, y=w1135) -> (x/y=w1140:dbl)
        n426 = Divide(x=w1123, y=w1117) -> (x/y=w1122:dbl)
        n427 = Divide(x=w1132, y=w1126) -> (x/y=w1131:dbl)
        n428 = To Double Precision Float(number=w1145) -> (double precision float=w1148:dbl)
        n429 = To Double Precision Float(number=w1118) -> (double precision float=w1121:dbl)
        n430 = Multiply(x=w1149, y=w1148) -> (x*y=w1147:dbl)
        n431 = Multiply(x=w1140, y=w1139) -> (x*y=w1138:dbl)
        n432 = Multiply(x=w1122, y=w1121) -> (x*y=w1120:dbl)
        n433 = Multiply(x=w1131, y=w1130) -> (x*y=w1129:dbl)
        n434 = To Long Integer(number=w1147) -> (32bit integer=w1146:i32)
        n435 = To Long Integer(number=w1138) -> (32bit integer=w1137:i32)
        n436 = To Long Integer(number=w1120) -> (32bit integer=w1119:i32)
        n437 = To Long Integer(number=w1129) -> (32bit integer=w1128:i32)
        n438 = property on="Reset Y Motor Steps" class="DigNum (strict)"("Val(Sgnl)"=w1146) -> ()  [unwired: 2 in, 2 out]
        n439 = property on="Reset X Motor Steps" class="DigNum (strict)"("Val(Sgnl)"=w1137) -> ()  [unwired: 2 in, 2 out]
        n440 = property on="Reset R Motor Steps" class="DigNum (strict)"("Val(Sgnl)"=w1119) -> ()  [unwired: 2 in, 2 out]
        n441 = property on="Reset Z Motor Steps" class="DigNum (strict)"("Val(Sgnl)"=w1128) -> ()  [unwired: 2 in, 2 out]
      }
      event "Y Velocity SP step/sec", "X Velocity SP step/sec", "R Velocity SP step/sec", "Z Velocity SP step/sec", "Y Step SP", "X Step SP", "Z Step SP", "R Step SP": Value Change {
        n442 = event-data() -> ()  [unwired: 1 in, 5 out]
        n443 = property on="X Step SP" class="DigNum (strict)"() -> ("Value"=w1176:i32)  [unwired: 2 in, 2 out]
        n444 = property on="Z Step SP" class="DigNum (strict)"() -> ("Value"=w1168:i32)  [unwired: 2 in, 2 out]
        n445 = property on="R Step SP" class="DigNum (strict)"() -> ("Value"=w1160:i32)  [unwired: 2 in, 2 out]
        n446 = property on="X offset mm" class="DigNum (strict)"() -> ("Value"=w1173:dbl)  [unwired: 2 in, 2 out]
        n447 = property on="Z offset mm" class="DigNum (strict)"() -> ("Value"=w1165:dbl)  [unwired: 2 in, 2 out]
        n448 = property on="R offset deg" class="DigNum (strict)"() -> ("Value"=w1157:dbl)  [unwired: 2 in, 2 out]
        n449 = property on="Y steps/rev" class="DigNum (strict)"() -> ("Value"=w1182:u32)  [unwired: 2 in, 2 out]
        n450 = property on="Y steps/rev" class="DigNum (strict)"() -> ("Value"=w1207:u32)  [unwired: 2 in, 2 out]
        n451 = property on="X steps/rev" class="DigNum (strict)"() -> ("Value"=w1174:u32)  [unwired: 2 in, 2 out]
        n452 = property on="X steps/rev" class="DigNum (strict)"() -> ("Value"=w1201:u32)  [unwired: 2 in, 2 out]
        n453 = property on="Z steps/rev" class="DigNum (strict)"() -> ("Value"=w1166:u32)  [unwired: 2 in, 2 out]
        n454 = property on="Z steps/rev" class="DigNum (strict)"() -> ("Value"=w1195:u32)  [unwired: 2 in, 2 out]
        n455 = property on="R steps/rev" class="DigNum (strict)"() -> ("Value"=w1158:u32)  [unwired: 2 in, 2 out]
        n456 = property on="R steps/rev" class="DigNum (strict)"() -> ("Value"=w1189:u32)  [unwired: 2 in, 2 out]
        n457 = property on="Y Step SP" class="DigNum (strict)"() -> ("Value"=w1184:i32)  [unwired: 2 in, 2 out]
        n458 = property on="Y Velocity SP step/sec" class="DigNum (strict)"() -> ("Value"=w1209:i32)  [unwired: 2 in, 2 out]
        n459 = property on="X Velocity SP step/sec" class="DigNum (strict)"() -> ("Value"=w1203:i32)  [unwired: 2 in, 2 out]
        n460 = property on="Z Velocity SP step/sec" class="DigNum (strict)"() -> ("Value"=w1197:i32)  [unwired: 2 in, 2 out]
        n461 = property on="R Velocity SP step/sec" class="DigNum (strict)"() -> ("Value"=w1191:i32)  [unwired: 2 in, 2 out]
        n462 = To Double Precision Float(number=w1184) -> (double precision float=w1185:dbl)
        n463 = To Double Precision Float(number=w1182) -> (double precision float=w1188:dbl)
        n464 = To Double Precision Float(number=w1207) -> (double precision float=w1212:dbl)
        n465 = To Double Precision Float(number=w1176) -> (double precision float=w1177:dbl)
        n466 = To Double Precision Float(number=w1174) -> (double precision float=w1180:dbl)
        n467 = To Double Precision Float(number=w1201) -> (double precision float=w1206:dbl)
        n468 = To Double Precision Float(number=w1168) -> (double precision float=w1169:dbl)
        n469 = To Double Precision Float(number=w1166) -> (double precision float=w1172:dbl)
        n470 = To Double Precision Float(number=w1195) -> (double precision float=w1200:dbl)
        n471 = To Double Precision Float(number=w1160) -> (double precision float=w1161:dbl)
        n472 = To Double Precision Float(number=w1158) -> (double precision float=w1164:dbl)
        n473 = To Double Precision Float(number=w1189) -> (double precision float=w1194:dbl)
        n474 = Divide(x=w1185, y=w1188) -> (x/y=w1187:dbl)
        n475 = Divide(x=w1177, y=w1180) -> (x/y=w1179:dbl)
        n476 = Divide(x=w1169, y=w1172) -> (x/y=w1171:dbl)
        n477 = Divide(x=w1161, y=w1164) -> (x/y=w1163:dbl)
        n478 = To Double Precision Float(number=w1209) -> (double precision float=w1210:dbl)
        n479 = To Double Precision Float(number=w1203) -> (double precision float=w1204:dbl)
        n480 = To Double Precision Float(number=w1197) -> (double precision float=w1198:dbl)
        n481 = To Double Precision Float(number=w1191) -> (double precision float=w1192:dbl)
        n482 = property on="Y mm/rev" class="DigNum (strict)"() -> ("Value"=w1153:dbl)  [unwired: 2 in, 2 out]
        n483 = property on="X mm/rev" class="DigNum (strict)"() -> ("Value"=w1154:dbl)  [unwired: 2 in, 2 out]
        n484 = property on="Z mm/rev" class="DigNum (strict)"() -> ("Value"=w1155:dbl)  [unwired: 2 in, 2 out]
        n485 = property on="R deg/rev" class="DigNum (strict)"() -> ("Value"=w1156:dbl)  [unwired: 2 in, 2 out]
        n486 = Multiply(x=w1187, y=w1153) -> (x*y=w1186:dbl)
        n487 = Divide(x=w1210, y=w1212) -> (x/y=w1211:dbl)
        n488 = Multiply(x=w1179, y=w1154) -> (x*y=w1178:dbl)
        n489 = Divide(x=w1204, y=w1206) -> (x/y=w1205:dbl)
        n490 = Multiply(x=w1171, y=w1155) -> (x*y=w1170:dbl)
        n491 = Divide(x=w1198, y=w1200) -> (x/y=w1199:dbl)
        n492 = Multiply(x=w1163, y=w1156) -> (x*y=w1162:dbl)
        n493 = Divide(x=w1192, y=w1194) -> (x/y=w1193:dbl)
        n494 = property on="Y offset mm" class="DigNum (strict)"() -> ("Value"=w1181:dbl)  [unwired: 2 in, 2 out]
        n495 = Add(x=w1186, y=w1181) -> (x+y=w1183:dbl)
        n496 = Multiply(x=w1211, y=w1153) -> (x*y=w1208:dbl)
        n497 = Add(x=w1178, y=w1173) -> (x+y=w1175:dbl)
        n498 = Multiply(x=w1205, y=w1154) -> (x*y=w1202:dbl)
        n499 = Add(x=w1170, y=w1165) -> (x+y=w1167:dbl)
        n500 = Multiply(x=w1199, y=w1155) -> (x*y=w1196:dbl)
        n501 = Add(x=w1162, y=w1157) -> (x+y=w1159:dbl)
        n502 = Multiply(x=w1193, y=w1156) -> (x*y=w1190:dbl)
        n503 = property on="Y Position MV mm" class="DigNum (strict)"("Val(Sgnl)"=w1183) -> ()  [unwired: 2 in, 2 out]
        n504 = property on="Y Velocity MV mm/sec" class="DigNum (strict)"("Val(Sgnl)"=w1208) -> ()  [unwired: 2 in, 2 out]
        n505 = property on="X Position MV mm" class="DigNum (strict)"("Val(Sgnl)"=w1175) -> ()  [unwired: 2 in, 2 out]
        n506 = property on="X Velocity MV mm/sec" class="DigNum (strict)"("Val(Sgnl)"=w1202) -> ()  [unwired: 2 in, 2 out]
        n507 = property on="Z Position MV mm" class="DigNum (strict)"("Val(Sgnl)"=w1167) -> ()  [unwired: 2 in, 2 out]
        n508 = property on="Z Velocity MV mm/sec" class="DigNum (strict)"("Val(Sgnl)"=w1196) -> ()  [unwired: 2 in, 2 out]
        n509 = property on="R Position MV deg" class="DigNum (strict)"("Val(Sgnl)"=w1159) -> ()  [unwired: 2 in, 2 out]
        n510 = Absolute Value(x=w1190) -> (abs(x)=w1152:dbl)
        n511 = property on="R Velocity MVdeg/sec" class="DigNum (strict)"("Val(Sgnl)"=w1152) -> ()  [unwired: 2 in, 2 out]
      }
      event "APX:MY_RQ": Value Change {
        n512 = event-data() -> ()  [unwired: 1 in, 6 out]
        n513 = flat-sequence {
          tunnel: w1217 -> [w1225]
          tunnel: w1218 -> [w1226]
          tunnel: [w1226] -> w1214
          tunnel: [w1225] -> w1213
          tunnel: [w1248] -> w1216
          tunnel: [w1247] -> w1215
          tunnel: w1214 -> [w1250]
          tunnel: w1213 -> [w1249]
          tunnel: [w1266] -> w1220
          tunnel: [w1265] -> w1219
          tunnel: w1216 -> [w1264]
          tunnel: w1215 -> [w1263]
          tunnel: [w1275] -> w1222
          tunnel: [w1274] -> w1221
          tunnel: w1220 -> [w1273]
          tunnel: w1219 -> [w1272]
          tunnel: [w1281] -> w1223
          tunnel: [w1282] -> w1224
          tunnel: w1222 -> [w1282]
          tunnel: w1221 -> [w1280]
          frame #0 {
            (unwired) T2."Disabled and Grayed Out" ("Disabled")
            (unwired) T2."Disabled and Grayed Out" ("Disabled")
            n514 = flat-sequence {
              frame #0 {
                n515 = property on="Y steps/rev" class="DigNum (strict)"() -> ("Value"=w1243:u32)  [unwired: 2 in, 2 out]
                n516 = property on="Y Velocity SP step/sec" class="DigNum (strict)"() -> ("Maximum"=w1230:dbl)  [unwired: 2 in, 2 out]
                n517 = property on="APX:MY_VLC_RQ" class="DigNum (strict)"() -> ("Value"=w1234:dbl)  [unwired: 2 in, 2 out]
                n518 = property on="Y Velocity SP step/sec" class="DigNum (strict)"() -> ("Minimum"=w1229:dbl)  [unwired: 2 in, 2 out]
                n519 = property on="APX:MY_RQ" class="DigNum (strict)"() -> ("Value"=w1240:dbl)  [unwired: 2 in, 2 out]
                n520 = property on="Y offset mm" class="DigNum (strict)"() -> ("Value"=w1241:dbl)  [unwired: 2 in, 2 out]
                n521 = property on="Y mm/rev" class="DigNum (strict)"() -> ("Value"=w1227:dbl)  [unwired: 2 in, 2 out]
                n522 = Divide(x=w1234, y=w1227) -> (x/y=w1235:dbl)
                n523 = Subtract(x=w1240, y=w1241) -> (x-y=w1244:dbl)
                n524 = To Double Precision Float(number=w1243) -> (double precision float=w1228:dbl)
                n525 = Multiply(x=w1235, y=w1228) -> (x*y=w1232:dbl)
                n526 = Divide(x=w1244, y=w1227) -> (x/y=w1245:dbl)
                n527 = property on="Y Step SP" class="DigNum (strict)"() -> ("Maximum"=w1237:dbl)  [unwired: 2 in, 2 out]
                n528 = property on="Y Step SP" class="DigNum (strict)"() -> ("Minimum"=w1236:dbl)  [unwired: 2 in, 2 out]
                n529 = In Range and Coerce(upper limit=w1230, x=w1232, lower limit=w1229) -> (coerced(x)=w1231:dbl)  [unwired: 1 out]
                n530 = Multiply(x=w1245, y=w1228) -> (x*y=w1239:dbl)
                n531 = In Range and Coerce(upper limit=w1237, x=w1239, lower limit=w1236) -> (coerced(x)=w1238:dbl)  [unwired: 1 out]
                n532 = To Long Integer(number=w1231) -> (32bit integer=w1233:i32)
                n533 = property on="Y Velocity SP step/sec" class="DigNum (strict)"("Val(Sgnl)"=w1233) -> ()  [unwired: 2 in, 2 out]
                n534 = To Long Integer(number=w1238) -> (32bit integer=w1242:i32)
                n535 = property on="Y Step SP" class="DigNum (strict)"("Val(Sgnl)"=w1242) -> ()  [unwired: 2 in, 2 out]
              }
            }
          }
          frame #1 {
            n536 = property on="Y Backlash" class="DigNum (strict)"() -> ("Value"=w1246:i32)  [unwired: 2 in, 2 out]
            n537 = property on="Y Step PV" class="DigNum (strict)"() -> ("Value"=w1257:i32)  [unwired: 2 in, 2 out]
            n538 = property on="Y Step SP" class="DigNum (strict)"() -> ("Value"=w1258:i32)  [unwired: 2 in, 2 out]
            n539 = Subtract(x=w1258, y=w1257) -> (x-y=w1256:i32)
            n540 = Sign(1:w1246) -> (0:w1254:i32)
            n541 = Sign(1:w1256) -> (0:w1255:i32)
            n542 = Multiply(x=w1255, y=w1254) -> (x*y=w1253:i32)
            n543 = Equal?(x=w1253, y=1) -> (x = y?=w1251:bool)
            n544 = case shown="True" w1251 {
              tunnel: w1250 -> [w1260 w1262]
              tunnel: w1249 -> [w1259 w1261]
              tunnel: [w1259 w1261] -> w1248
              tunnel: [w1260 w1262] -> w1247
              frame False {
                (unwired) FALSE ("Value (Signaling)")
              }
              frame True {
                (unwired) TRUE ("Value (Signaling)")
              }
            }
          }
          frame #2 {
            # "Velocity Setting"
            n545 = property on="Y Velocity SP step/sec" class="DigNum (strict)"() -> ("Value"=w1267:i32)  [unwired: 2 in, 2 out]
            n546 = Number To Decimal String(number=w1267) -> (decimal integer string=w1268:string)  [unwired: 1 in]
            n547 = call "mDrive Send Command.vi"("error in (no error)"=w1264, "Extra"=w1268, "Command"=T1."Max Velocity", "VISA resource name"=w1263) -> ("error out"=w1265:errorcluster, "VISA resource name out"=w1266:refnum<visa-resource-name>)  [unwired: 3 in, 1 out]
          }
          frame #3 {
            # "Move to Abs Position"
            n548 = call "Time Delay5"("error in (no error)"=w1272, "Delay Time (s)"=0.5) -> ("error out"=w1271:errorcluster)  [unwired: 9 in]
            n549 = property on="Y Step SP" class="DigNum (strict)"() -> ("Value"=w1278:i32)  [unwired: 2 in, 2 out]
            n550 = Number To Decimal String(number=w1278) -> (decimal integer string=w1277:string)  [unwired: 1 in]
            n551 = call "mDrive Send Command.vi"("error in (no error)"=w1271, "Extra"=w1277, "Command"=T1."Move to Absolute Position", "VISA resource name"=w1273) -> ("error out"=w1274:errorcluster, "VISA resource name out"=w1275:refnum<visa-resource-name>)  [unwired: 3 in, 1 out]
          }
          frame #4 {
            n552 = call "Time Delay"("error in (no error)"=w1280, "Delay Time (s)"=0.3) -> ("error out"=w1281:errorcluster)  [unwired: 9 in]
          }
        }
      }
      event "APX:MZ_RQ": Value Change {
        n553 = event-data() -> ()  [unwired: 1 in, 6 out]
        n554 = flat-sequence {
          tunnel: w1285 -> [w1295]
          tunnel: w1286 -> [w1296]
          tunnel: [w1296] -> w1288
          tunnel: [w1295] -> w1287
          tunnel: [w1318] -> w1290
          tunnel: [w1317] -> w1289
          tunnel: w1288 -> [w1320]
          tunnel: w1287 -> [w1319]
          tunnel: [w1336] -> w1292
          tunnel: [w1335] -> w1291
          tunnel: w1290 -> [w1334]
          tunnel: w1289 -> [w1333]
          tunnel: [w1344] -> w1294
          tunnel: [w1343] -> w1293
          tunnel: w1292 -> [w1342]
          tunnel: w1291 -> [w1341]
          tunnel: [w1350] -> w1284
          tunnel: [w1351] -> w1283
          tunnel: w1294 -> [w1351]
          tunnel: w1293 -> [w1349]
          frame #0 {
            (unwired) T2."Disabled and Grayed Out" ("Disabled")
            (unwired) T2."Disabled and Grayed Out" ("Disabled")
            n555 = flat-sequence {
              frame #0 {
                n556 = property on="Z steps/rev" class="DigNum (strict)"() -> ("Value"=w1311:u32)  [unwired: 2 in, 2 out]
                n557 = property on="Z Velocity SP step/sec" class="DigNum (strict)"() -> ("Maximum"=w1298:dbl)  [unwired: 2 in, 2 out]
                n558 = property on="APX:MZ_VLC_RQ" class="DigNum (strict)"() -> ("Value"=w1302:dbl)  [unwired: 2 in, 2 out]
                n559 = property on="Z Velocity SP step/sec" class="DigNum (strict)"() -> ("Minimum"=w1297:dbl)  [unwired: 2 in, 2 out]
                n560 = property on="APX:MZ_RQ" class="DigNum (strict)"() -> ("Value"=w1308:dbl)  [unwired: 2 in, 2 out]
                n561 = property on="Z offset mm" class="DigNum (strict)"() -> ("Value"=w1309:dbl)  [unwired: 2 in, 2 out]
                n562 = property on="Z mm/rev" class="DigNum (strict)"() -> ("Value"=w1314:dbl)  [unwired: 2 in, 2 out]
                n563 = Divide(x=w1302, y=w1314) -> (x/y=w1303:dbl)
                n564 = Subtract(x=w1308, y=w1309) -> (x-y=w1312:dbl)
                n565 = To Double Precision Float(number=w1311) -> (double precision float=w1315:dbl)
                n566 = Multiply(x=w1303, y=w1315) -> (x*y=w1300:dbl)
                n567 = Divide(x=w1312, y=w1314) -> (x/y=w1313:dbl)
                n568 = property on="Z Step SP" class="DigNum (strict)"() -> ("Maximum"=w1305:dbl)  [unwired: 2 in, 2 out]
                n569 = property on="Z Step SP" class="DigNum (strict)"() -> ("Minimum"=w1304:dbl)  [unwired: 2 in, 2 out]
                n570 = In Range and Coerce(upper limit=w1298, x=w1300, lower limit=w1297) -> (coerced(x)=w1299:dbl)  [unwired: 1 out]
                n571 = Multiply(x=w1313, y=w1315) -> (x*y=w1307:dbl)
                n572 = In Range and Coerce(upper limit=w1305, x=w1307, lower limit=w1304) -> (coerced(x)=w1306:dbl)  [unwired: 1 out]
                n573 = To Long Integer(number=w1299) -> (32bit integer=w1301:i32)
                n574 = property on="Z Velocity SP step/sec" class="DigNum (strict)"("Val(Sgnl)"=w1301) -> ()  [unwired: 2 in, 2 out]
                n575 = To Long Integer(number=w1306) -> (32bit integer=w1310:i32)
                n576 = property on="Z Step SP" class="DigNum (strict)"("Val(Sgnl)"=w1310) -> ()  [unwired: 2 in, 2 out]
              }
            }
          }
          frame #1 {
            n577 = property on="Z Backlash" class="DigNum (strict)"() -> ("Value"=w1316:i32)  [unwired: 2 in, 2 out]
            n578 = property on="Z Step PV" class="DigNum (strict)"() -> ("Value"=w1327:i32)  [unwired: 2 in, 2 out]
            n579 = property on="Z Step SP" class="DigNum (strict)"() -> ("Value"=w1328:i32)  [unwired: 2 in, 2 out]
            n580 = Subtract(x=w1328, y=w1327) -> (x-y=w1326:i32)
            n581 = Sign(1:w1316) -> (0:w1324:i32)
            n582 = Sign(1:w1326) -> (0:w1325:i32)
            n583 = Multiply(x=w1325, y=w1324) -> (x*y=w1323:i32)
            n584 = Equal?(x=w1323, y=1) -> (x = y?=w1321:bool)
            n585 = case shown="True" w1321 {
              tunnel: w1320 -> [w1330 w1332]
              tunnel: w1319 -> [w1329 w1331]
              tunnel: [w1329 w1331] -> w1318
              tunnel: [w1330 w1332] -> w1317
              frame False {
                (unwired) FALSE ("Value (Signaling)")
              }
              frame True {
                (unwired) TRUE ("Value (Signaling)")
              }
            }
          }
          frame #2 {
            # "Velocity Setting"
            n586 = property on="Z Velocity SP step/sec" class="DigNum (strict)"() -> ("Value"=w1337:i32)  [unwired: 2 in, 2 out]
            n587 = Number To Decimal String(number=w1337) -> (decimal integer string=w1338:string)  [unwired: 1 in]
            n588 = call "mDrive Send Command.vi"("error in (no error)"=w1334, "Extra"=w1338, "Command"=T1."Max Velocity", "VISA resource name"=w1333) -> ("error out"=w1335:errorcluster, "VISA resource name out"=w1336:refnum<visa-resource-name>)  [unwired: 3 in, 1 out]
          }
          frame #3 {
            # "Move to Abs Position"
            n589 = call "Time Delay7"("error in (no error)"=w1341) -> ("error out"=w1340:errorcluster)  [unwired: 10 in]
            n590 = property on="Z Step SP" class="DigNum (strict)"() -> ("Value"=w1347:i32)  [unwired: 2 in, 2 out]
            n591 = Number To Decimal String(number=w1347) -> (decimal integer string=w1346:string)  [unwired: 1 in]
            n592 = call "mDrive Send Command.vi"("error in (no error)"=w1340, "Extra"=w1346, "Command"=T1."Move to Absolute Position", "VISA resource name"=w1342) -> ("error out"=w1343:errorcluster, "VISA resource name out"=w1344:refnum<visa-resource-name>)  [unwired: 3 in, 1 out]
          }
          frame #4 {
            n593 = call "Time Delay28"("error in (no error)"=w1349, "Delay Time (s)"=0.1) -> ("error out"=w1350:errorcluster)  [unwired: 9 in]
          }
        }
      }
      event "APX:MR_RQ": Value Change {
        n594 = event-data() -> ()  [unwired: 1 in, 6 out]
        n595 = flat-sequence {
          tunnel: w1354 -> [w1364]
          tunnel: w1355 -> [w1365]
          tunnel: [w1365] -> w1357
          tunnel: [w1364] -> w1356
          tunnel: [w1388] -> w1359
          tunnel: [w1387] -> w1358
          tunnel: w1357 -> [w1390]
          tunnel: w1356 -> [w1389]
          tunnel: [w1406] -> w1361
          tunnel: [w1405] -> w1360
          tunnel: w1359 -> [w1404]
          tunnel: w1358 -> [w1403]
          tunnel: [w1413] -> w1363
          tunnel: [w1412] -> w1362
          tunnel: w1361 -> [w1411]
          tunnel: w1360 -> [w1410]
          tunnel: [w1419] -> w1353
          tunnel: [w1420] -> w1352
          tunnel: w1363 -> [w1420]
          tunnel: w1362 -> [w1418]
          frame #0 {
            (unwired) T2."Disabled and Grayed Out" ("Disabled")
            (unwired) T2."Disabled and Grayed Out" ("Disabled")
            n596 = flat-sequence {
              frame #0 {
                n597 = property on="R steps/rev" class="DigNum (strict)"() -> ("Value"=w1383:u32)  [unwired: 2 in, 2 out]
                n598 = property on="R Velocity SP step/sec" class="DigNum (strict)"() -> ("Maximum"=w1370:dbl)  [unwired: 2 in, 2 out]
                n599 = property on="R Velocity SP step/sec" class="DigNum (strict)"() -> ("Minimum"=w1369:dbl)  [unwired: 2 in, 2 out]
                n600 = property on="APX:MR_VLC_RQ" class="DigNum (strict)"() -> ("Value"=w1374:dbl)  [unwired: 2 in, 2 out]
                n601 = property on="APX:MR_RQ" class="DigNum (strict)"() -> ("Value"=w1380:dbl)  [unwired: 2 in, 2 out]
                n602 = property on="R offset deg" class="DigNum (strict)"() -> ("Value"=w1381:dbl)  [unwired: 2 in, 2 out]
                n603 = property on="R deg/rev" class="DigNum (strict)"() -> ("Value"=w1367:dbl)  [unwired: 2 in, 2 out]
                n604 = Divide(x=w1374, y=w1367) -> (x/y=w1375:dbl)
                n605 = Subtract(x=w1380, y=w1381) -> (x-y=w1384:dbl)
                n606 = To Double Precision Float(number=w1383) -> (double precision float=w1368:dbl)
                n607 = Multiply(x=w1375, y=w1368) -> (x*y=w1372:dbl)
                n608 = Divide(x=w1384, y=w1367) -> (x/y=w1385:dbl)
                n609 = property on="R Step SP" class="DigNum (strict)"() -> ("Maximum"=w1377:dbl)  [unwired: 2 in, 2 out]
                n610 = property on="R Step SP" class="DigNum (strict)"() -> ("Minimum"=w1376:dbl)  [unwired: 2 in, 2 out]
                n611 = Multiply(x=w1385, y=w1368) -> (x*y=w1379:dbl)
                n612 = Absolute Value(x=w1372) -> (abs(x)=w1366:dbl)
                n613 = In Range and Coerce(upper limit=w1370, x=w1366, lower limit=w1369) -> (coerced(x)=w1371:dbl)  [unwired: 1 out]
                n614 = In Range and Coerce(upper limit=w1377, x=w1379, lower limit=w1376) -> (coerced(x)=w1378:dbl)  [unwired: 1 out]
                n615 = To Long Integer(number=w1371) -> (32bit integer=w1373:i32)
                n616 = To Long Integer(number=w1378) -> (32bit integer=w1382:i32)
                n617 = property on="R Velocity SP step/sec" class="DigNum (strict)"("Val(Sgnl)"=w1373) -> ()  [unwired: 2 in, 2 out]
                n618 = property on="R Step SP" class="DigNum (strict)"("Val(Sgnl)"=w1382) -> ()  [unwired: 2 in, 2 out]
              }
            }
          }
          frame #1 {
            n619 = property on="R Backlash" class="DigNum (strict)"() -> ("Value"=w1386:i32)  [unwired: 2 in, 2 out]
            n620 = property on="R Step PV" class="DigNum (strict)"() -> ("Value"=w1397:i32)  [unwired: 2 in, 2 out]
            n621 = property on="R Step SP" class="DigNum (strict)"() -> ("Value"=w1398:i32)  [unwired: 2 in, 2 out]
            n622 = Subtract(x=w1398, y=w1397) -> (x-y=w1396:i32)
            n623 = Sign(1:w1386) -> (0:w1394:i32)
            n624 = Sign(1:w1396) -> (0:w1395:i32)
            n625 = Multiply(x=w1395, y=w1394) -> (x*y=w1393:i32)
            n626 = Equal?(x=w1393, y=1) -> (x = y?=w1391:bool)
            n627 = case shown="True" w1391 {
              tunnel: w1390 -> [w1400 w1402]
              tunnel: w1389 -> [w1399 w1401]
              tunnel: [w1399 w1401] -> w1388
              tunnel: [w1400 w1402] -> w1387
              frame False {
                (unwired) FALSE ("Value (Signaling)")
              }
              frame True {
                (unwired) TRUE ("Value (Signaling)")
              }
            }
          }
          frame #2 {
            # "Velocity Setting"
            n628 = property on="R Velocity SP step/sec" class="DigNum (strict)"() -> ("Value"=w1407:i32)  [unwired: 2 in, 2 out]
            n629 = Number To Decimal String(number=w1407) -> (decimal integer string=w1408:string)  [unwired: 1 in]
            n630 = call "mDrive Send Command.vi"("error in (no error)"=w1404, "Extra"=w1408, "Command"=T1."Max Velocity", "VISA resource name"=w1403) -> ("error out"=w1405:errorcluster, "VISA resource name out"=w1406:refnum<visa-resource-name>)  [unwired: 3 in, 1 out]
          }
          frame #3 {
            # "Move to Abs Position"
            n631 = property on="R Step SP" class="DigNum (strict)"() -> ("Value"=w1416:i32)  [unwired: 2 in, 2 out]
            n632 = Number To Decimal String(number=w1416) -> (decimal integer string=w1415:string)  [unwired: 1 in]
            n633 = call "mDrive Send Command.vi"("error in (no error)"=w1410, "Extra"=w1415, "Command"=T1."Move to Absolute Position", "VISA resource name"=w1411) -> ("error out"=w1412:errorcluster, "VISA resource name out"=w1413:refnum<visa-resource-name>)  [unwired: 3 in, 1 out]
          }
          frame #4 {
            n634 = call "Time Delay29"("error in (no error)"=w1418, "Delay Time (s)"=0.1) -> ("error out"=w1419:errorcluster)  [unwired: 9 in]
          }
        }
      }
      event "APX:MX_RQ": Value Change {
        n635 = event-data() -> ()  [unwired: 1 in, 6 out]
        n636 = flat-sequence {
          tunnel: [w1434] -> w1426
          tunnel: [w1433] -> w1425
          tunnel: w1424 -> [w1434]
          tunnel: w1423 -> [w1433]
          tunnel: [w1456] -> w1428
          tunnel: [w1455] -> w1427
          tunnel: w1426 -> [w1458]
          tunnel: w1425 -> [w1457]
          tunnel: [w1474] -> w1430
          tunnel: [w1473] -> w1429
          tunnel: w1428 -> [w1472]
          tunnel: w1427 -> [w1471]
          tunnel: [w1482] -> w1432
          tunnel: [w1481] -> w1431
          tunnel: w1430 -> [w1480]
          tunnel: w1429 -> [w1479]
          tunnel: [w1488] -> w1421
          tunnel: [w1489] -> w1422
          tunnel: w1432 -> [w1489]
          tunnel: w1431 -> [w1487]
          frame #0 {
            (unwired) T2."Disabled and Grayed Out" ("Disabled")
            (unwired) T2."Disabled and Grayed Out" ("Disabled")
            n637 = flat-sequence {
              frame #0 {
                n638 = property on="X steps/rev" class="DigNum (strict)"() -> ("Value"=w1451:u32)  [unwired: 2 in, 2 out]
                n639 = property on="X Velocity SP step/sec" class="DigNum (strict)"() -> ("Maximum"=w1438:dbl)  [unwired: 2 in, 2 out]
                n640 = property on="APX:MX_VLC_RQ" class="DigNum (strict)"() -> ("Value"=w1442:dbl)  [unwired: 2 in, 2 out]
                n641 = property on="X Velocity SP step/sec" class="DigNum (strict)"() -> ("Minimum"=w1437:dbl)  [unwired: 2 in, 2 out]
                n642 = property on="APX:MX_RQ" class="DigNum (strict)"() -> ("Value"=w1448:dbl)  [unwired: 2 in, 2 out]
                n643 = property on="X offset mm" class="DigNum (strict)"() -> ("Value"=w1449:dbl)  [unwired: 2 in, 2 out]
                n644 = property on="X mm/rev" class="DigNum (strict)"() -> ("Value"=w1435:dbl)  [unwired: 2 in, 2 out]
                n645 = Divide(x=w1442, y=w1435) -> (x/y=w1443:dbl)
                n646 = Subtract(x=w1448, y=w1449) -> (x-y=w1452:dbl)
                n647 = To Double Precision Float(number=w1451) -> (double precision float=w1436:dbl)
                n648 = Multiply(x=w1443, y=w1436) -> (x*y=w1440:dbl)
                n649 = Divide(x=w1452, y=w1435) -> (x/y=w1453:dbl)
                n650 = property on="X Step SP" class="DigNum (strict)"() -> ("Maximum"=w1445:dbl)  [unwired: 2 in, 2 out]
                n651 = property on="X Step SP" class="DigNum (strict)"() -> ("Minimum"=w1444:dbl)  [unwired: 2 in, 2 out]
                n652 = Multiply(x=w1453, y=w1436) -> (x*y=w1447:dbl)
                n653 = In Range and Coerce(upper limit=w1438, x=w1440, lower limit=w1437) -> (coerced(x)=w1439:dbl)  [unwired: 1 out]
                n654 = In Range and Coerce(upper limit=w1445, x=w1447, lower limit=w1444) -> (coerced(x)=w1446:dbl)  [unwired: 1 out]
                n655 = To Long Integer(number=w1439) -> (32bit integer=w1441:i32)
                n656 = property on="X Velocity SP step/sec" class="DigNum (strict)"("Val(Sgnl)"=w1441) -> ()  [unwired: 2 in, 2 out]
                n657 = To Long Integer(number=w1446) -> (32bit integer=w1450:i32)
                n658 = property on="X Step SP" class="DigNum (strict)"("Val(Sgnl)"=w1450) -> ()  [unwired: 2 in, 2 out]
              }
            }
          }
          frame #1 {
            n659 = property on="X Backlash" class="DigNum (strict)"() -> ("Value"=w1454:i32)  [unwired: 2 in, 2 out]
            n660 = property on="X Step PV" class="DigNum (strict)"() -> ("Value"=w1465:i32)  [unwired: 2 in, 2 out]
            n661 = property on="X Step SP" class="DigNum (strict)"() -> ("Value"=w1466:i32)  [unwired: 2 in, 2 out]
            n662 = Subtract(x=w1466, y=w1465) -> (x-y=w1464:i32)
            n663 = Sign(1:w1454) -> (0:w1462:i32)
            n664 = Sign(1:w1464) -> (0:w1463:i32)
            n665 = Multiply(x=w1463, y=w1462) -> (x*y=w1461:i32)
            n666 = Equal?(x=w1461, y=1) -> (x = y?=w1459:bool)
            n667 = case shown="True" w1459 {
              tunnel: w1458 -> [w1468 w1470]
              tunnel: w1457 -> [w1467 w1469]
              tunnel: [w1467 w1469] -> w1456
              tunnel: [w1468 w1470] -> w1455
              frame False {
                (unwired) FALSE ("Value (Signaling)")
              }
              frame True {
                (unwired) TRUE ("Value (Signaling)")
              }
            }
          }
          frame #2 {
            # "Velocity Setting"
            n668 = property on="X Velocity SP step/sec" class="DigNum (strict)"() -> ("Value"=w1475:i32)  [unwired: 2 in, 2 out]
            n669 = Number To Decimal String(number=w1475) -> (decimal integer string=w1476:string)  [unwired: 1 in]
            n670 = call "mDrive Send Command.vi"("error in (no error)"=w1472, "Extra"=w1476, "Command"=T1."Max Velocity", "VISA resource name"=w1471) -> ("error out"=w1473:errorcluster, "VISA resource name out"=w1474:refnum<visa-resource-name>)  [unwired: 3 in, 1 out]
          }
          frame #3 {
            # "Move to Abs Position"
            n671 = call "Time Delay6"("error in (no error)"=w1479) -> ("error out"=w1478:errorcluster)  [unwired: 10 in]
            n672 = property on="X Step SP" class="DigNum (strict)"() -> ("Value"=w1485:i32)  [unwired: 2 in, 2 out]
            n673 = Number To Decimal String(number=w1485) -> (decimal integer string=w1484:string)  [unwired: 1 in]
            n674 = call "mDrive Send Command.vi"("error in (no error)"=w1478, "Extra"=w1484, "Command"=T1."Move to Absolute Position", "VISA resource name"=w1480) -> ("error out"=w1481:errorcluster, "VISA resource name out"=w1482:refnum<visa-resource-name>)  [unwired: 3 in, 1 out]
          }
          frame #4 {
            n675 = call "Time Delay15"("error in (no error)"=w1487, "Delay Time (s)"=0.1) -> ("error out"=w1488:errorcluster)  [unwired: 9 in]
          }
        }
      }
      event "APX:MXYZR_STOP": Mouse Down {
        n676 = event-data() -> ()  [unwired: 1 in, 7 out]
        n677 = flat-sequence {
          tunnel: [w1519] -> w1501
          tunnel: [w1518] -> w1500
          tunnel: w1499 -> [w1517]
          tunnel: w1498 -> [w1516]
          frame #0 {
            n678 = call "mDrive Send Command.vi"("error in (no error)"=w1516, "Command"=T1."Stop", "VISA resource name"=w1517) -> ("error out"=w1518:errorcluster, "VISA resource name out"=w1519:refnum<visa-resource-name>)  [unwired: 4 in, 1 out]
          }
        }
        n679 = flat-sequence {
          tunnel: w1505 -> [w1525]
          tunnel: w1504 -> [w1524]
          tunnel: [w1523] -> w1503
          tunnel: [w1522] -> w1502
          frame #0 {
            n680 = call "mDrive Send Command.vi"("error in (no error)"=w1524, "Command"=T1."Stop", "VISA resource name"=w1525) -> ("error out"=w1522:errorcluster, "VISA resource name out"=w1523:refnum<visa-resource-name>)  [unwired: 4 in, 1 out]
          }
        }
        n681 = flat-sequence {
          tunnel: [w1514] -> w1495
          tunnel: [w1513] -> w1494
          tunnel: w1497 -> [w1512]
          tunnel: w1496 -> [w1511]
          frame #0 {
            n682 = call "mDrive Send Command.vi"("error in (no error)"=w1511, "Command"=T1."Stop", "VISA resource name"=w1512) -> ("error out"=w1513:errorcluster, "VISA resource name out"=w1514:refnum<visa-resource-name>)  [unwired: 4 in, 1 out]
          }
        }
        n683 = flat-sequence {
          tunnel: w1493 -> [w1510]
          tunnel: w1492 -> [w1509]
          tunnel: [w1508] -> w1491
          tunnel: [w1506] -> _
          tunnel: [w1506] -> w1490
          frame #0 {
            n684 = call "mDrive Send Command.vi"("error in (no error)"=w1509, "Command"=T1."Stop", "VISA resource name"=w1510) -> ("error out"=w1506:errorcluster, "VISA resource name out"=w1508:refnum<visa-resource-name>)  [unwired: 4 in, 1 out]
          }
        }
      }
      event "Reset": Mouse Down {
        n685 = event-data() -> ()  [unwired: 1 in, 7 out]
        n686 = flat-sequence {
          tunnel: [w1556] -> w1535
          tunnel: w1536 -> [w1559]
          tunnel: [w1558] -> w1534
          tunnel: w1537 -> [w1557]
          frame #0 {
            n687 = property on="Reset X Motor Steps" class="DigNum (strict)"() -> ("Value"=w1560:i32)  [unwired: 2 in, 2 out]
            n688 = Number To Decimal String(number=w1560) -> (decimal integer string=w1561:string)  [unwired: 1 in]
            n689 = call "mDrive Send Command.vi"("error in (no error)"=w1559, "Extra"=w1561, "Command"=T1."Set Current Position", "VISA resource name"=w1557) -> ("error out"=w1558:errorcluster, "VISA resource name out"=w1556:refnum<visa-resource-name>)  [unwired: 3 in, 1 out]
          }
        }
        n690 = flat-sequence {
          tunnel: w1541 -> [w1566]
          tunnel: w1540 -> [w1565]
          tunnel: [w1564] -> w1539
          tunnel: [w1563] -> w1538
          frame #0 {
            n691 = property on="Reset Y Motor Steps" class="DigNum (strict)"() -> ("Value"=w1567:i32)  [unwired: 2 in, 2 out]
            n692 = Number To Decimal String(number=w1567) -> (decimal integer string=w1568:string)  [unwired: 1 in]
            n693 = call "mDrive Send Command.vi"("error in (no error)"=w1565, "Extra"=w1568, "Command"=T1."Set Current Position", "VISA resource name"=w1566) -> ("error out"=w1563:errorcluster, "VISA resource name out"=w1564:refnum<visa-resource-name>)  [unwired: 3 in, 1 out]
          }
        }
        n694 = flat-sequence {
          tunnel: [w1543] -> w1529
          tunnel: [w1545] -> w1528
          tunnel: w1531 -> [w1544]
          tunnel: w1530 -> [w1542]
          frame #0 {
            n695 = property on="Reset R Motor Steps" class="DigNum (strict)"() -> ("Value"=w1546:i32)  [unwired: 2 in, 2 out]
            n696 = Number To Decimal String(number=w1546) -> (decimal integer string=w1547:string)  [unwired: 1 in]
            n697 = call "mDrive Send Command.vi"("error in (no error)"=w1542, "Extra"=w1547, "Command"=T1."Set Current Position", "VISA resource name"=w1544) -> ("error out"=w1545:errorcluster, "VISA resource name out"=w1543:refnum<visa-resource-name>)  [unwired: 3 in, 1 out]
          }
        }
        n698 = flat-sequence {
          tunnel: [w1552] -> w1527
          tunnel: [w1551] -> w1526
          tunnel: w1533 -> [w1550]
          tunnel: w1532 -> [w1549]
          frame #0 {
            n699 = property on="Reset Z Motor Steps" class="DigNum (strict)"() -> ("Value"=w1553:i32)  [unwired: 2 in, 2 out]
            n700 = Number To Decimal String(number=w1553) -> (decimal integer string=w1554:string)  [unwired: 1 in]
            n701 = call "mDrive Send Command.vi"("error in (no error)"=w1549, "Extra"=w1554, "Command"=T1."Set Current Position", "VISA resource name"=w1550) -> ("error out"=w1551:errorcluster, "VISA resource name out"=w1552:refnum<visa-resource-name>)  [unwired: 3 in, 1 out]
          }
        }
      }
    }
    n702 = property on="Preset positions" class="Ring (strict)"() -> ("Strings []"=w443:string[])  [unwired: 2 in, 2 out]
    n703 = case shown="True" "Set Button" {
      tunnel: "Preset positions" -> [_ w493]
      frame False {
      }
      frame True {
        n704 = property on="Presets" class="Arr (strict)"() -> ("Value"=w490:i32[][])  [unwired: 2 in, 2 out]
        n705 = Index Array(array=w490, index (row)=w493) -> (element=w492:i32[])  [unwired: 1 in]
        n706 = Array To Cluster(array=w492) -> (cluster=w491:T4)
        n707 = Unbundle(w491) -> ("Value[0]"=w489:i32, "Value[1]"=w488:i32, "Value[2]"=w487:i32, "Value[3]"=w486:i32)  [unwired: 5 out]
        n708 = property on="X Step SP" class="DigNum (strict)"("Val(Sgnl)"=w489) -> ()  [unwired: 2 in, 2 out]
        n709 = property on="Y Step SP" class="DigNum (strict)"("Val(Sgnl)"=w488) -> ()  [unwired: 2 in, 2 out]
        n710 = property on="Z Step SP" class="DigNum (strict)"("Val(Sgnl)"=w487) -> ()  [unwired: 2 in, 2 out]
        n711 = property on="R Step SP" class="DigNum (strict)"("Val(Sgnl)"=w486) -> ()  [unwired: 2 in, 2 out]
      }
    }
    n712 = case shown="True" "Add Button" {
      tunnel: w443 -> [_ w485]
      frame False {
      }
      frame True {
        n713 = property on="X Step PV" class="DigNum (strict)"() -> ("Value"=w480:i32)  [unwired: 2 in, 2 out]
        n714 = property on="Y Step PV" class="DigNum (strict)"() -> ("Value"=w479:i32)  [unwired: 2 in, 2 out]
        n715 = property on="Z Step PV" class="DigNum (strict)"() -> ("Value"=w478:i32)  [unwired: 2 in, 2 out]
        n716 = property on="R Step PV" class="DigNum (strict)"() -> ("Value"=w477:i32)  [unwired: 2 in, 2 out]
        n717 = Build Array(w480, w479, w478, w477) -> (w483:i32[])
        n718 = Build Array (concatenate)(w485, "String") -> (w484:string[])
        n719 = property on="Preset positions" class="Ring (strict)"("Strings []"=w484) -> ()  [unwired: 2 in, 2 out]
        n720 = property on="Presets" class="Arr (strict)"() -> ("Value"=w482:i32[][])  [unwired: 2 in, 2 out]
        n721 = Build Array (concatenate)(w482, w483) -> (w476:i32[][])
        n722 = property on="Presets" class="Arr (strict)"("Val(Sgnl)"=w476) -> ()  [unwired: 2 in, 2 out]
      }
    }
    n723 = case shown="True" "Delete Button" {
      tunnel: w443 -> [_ w475]
      frame False {
      }
      frame True {
        n724 = property on="Preset positions" class="Ring (strict)"() -> ("Value"=w473:i32)  [unwired: 2 in, 2 out]
        n725 = Delete From Array(array=w475, index=w473) -> (array with subset deleted=w474:string[])  [unwired: 1 in, 1 out]
        n726 = property on="Presets" class="Arr (strict)"() -> ("Value"=w472:i32[][])  [unwired: 2 in, 2 out]
        n727 = property on="Preset positions" class="Ring (strict)"("Strings []"=w474) -> ()  [unwired: 2 in, 2 out]
        n728 = Delete From Array(array=w472, index (row)=w473) -> (array with subset deleted=w471:i32[][])  [unwired: 2 in, 1 out]
        n729 = property on="Presets" class="Arr (strict)"("Val(Sgnl)"=w471) -> ()  [unwired: 2 in, 2 out]
      }
    }
  }
  n730 = flat-sequence {
    tunnel: w88 -> [w1576]
    tunnel: w87 -> [w1574]
    tunnel: [w1571] -> w24
    frame #0 {
      n731 = call "mDrive Send Command.vi"("error in (no error)"=w1574, "Extra"="P", "Command"=T1."Print Parameter", "VISA resource name"=w1576) -> ("error out"=w1573:errorcluster, "read buffer"=w1580:string, "VISA resource name out"=w1575:refnum<visa-resource-name>)  [unwired: 3 in]
      n732 = call "Time Delay30"("error in (no error)"=w1573) -> ("error out"=w1570:errorcluster)  [unwired: 10 in]
      n733 = call "mDrive Send Command.vi"("error in (no error)"=w1570, "Command"=T1."Stop", "VISA resource name"=w1575) -> ("error out"=w1582:errorcluster, "VISA resource name out"=w1583:refnum<visa-resource-name>)  [unwired: 4 in, 1 out]
      n734 = Decimal String To Number(string=w1580, offset=0) -> (number=w1572:i32)  [unwired: 1 in, 1 out]
      n735 = To Long Integer(number=w1572) -> (32bit integer=w1571:i32)
      n736 = VISA Close(VISA resource name=w1583, error in (no error)=w1582) -> ()  [unwired: 1 out]
    }
  }
  n737 = flat-sequence {
    tunnel: w28 -> [w1590]
    tunnel: w27 -> [w1588]
    tunnel: [w1586] -> w23
    frame #0 {
      n738 = call "mDrive Send Command.vi"("error in (no error)"=w1588, "Extra"="P", "Command"=T1."Print Parameter", "VISA resource name"=w1590) -> ("error out"=w1585:errorcluster, "read buffer"=w1594:string, "VISA resource name out"=w1589:refnum<visa-resource-name>)  [unwired: 3 in]
      n739 = Decimal String To Number(string=w1594, offset=0) -> (number=w1587:i32)  [unwired: 1 in, 1 out]
      n740 = To Long Integer(number=w1587) -> (32bit integer=w1586:i32)
      n741 = call "Time Delay31"("error in (no error)"=w1585) -> ("error out"=w1584:errorcluster)  [unwired: 10 in]
      n742 = call "mDrive Send Command.vi"("error in (no error)"=w1584, "Command"=T1."Stop", "VISA resource name"=w1589) -> ("error out"=w1596:errorcluster, "VISA resource name out"=w1597:refnum<visa-resource-name>)  [unwired: 4 in, 1 out]
      n743 = VISA Close(VISA resource name=w1597, error in (no error)=w1596) -> ()  [unwired: 1 out]
    }
  }
  n744 = flat-sequence {
    tunnel: w30 -> [w1604]
    tunnel: w29 -> [w1602]
    tunnel: [w1599] -> w22
    frame #0 {
      n745 = call "mDrive Send Command.vi"("error in (no error)"=w1602, "Extra"="P", "Command"=T1."Print Parameter", "VISA resource name"=w1604) -> ("error out"=w1601:errorcluster, "read buffer"=w1608:string, "VISA resource name out"=w1603:refnum<visa-resource-name>)  [unwired: 3 in]
      n746 = call "Time Delay32"("error in (no error)"=w1601) -> ("error out"=w1598:errorcluster)  [unwired: 10 in]
      n747 = call "mDrive Send Command.vi"("error in (no error)"=w1598, "Command"=T1."Stop", "VISA resource name"=w1603) -> ("error out"=w1610:errorcluster, "VISA resource name out"=w1611:refnum<visa-resource-name>)  [unwired: 4 in, 1 out]
      n748 = Decimal String To Number(string=w1608, offset=0) -> (number=w1600:i32)  [unwired: 1 in, 1 out]
      n749 = To Long Integer(number=w1600) -> (32bit integer=w1599:i32)
      n750 = VISA Close(VISA resource name=w1611, error in (no error)=w1610) -> ()  [unwired: 1 out]
    }
  }
  n751 = flat-sequence {
    tunnel: w26 -> [w1618]
    tunnel: w25 -> [w1616]
    tunnel: [w1613] -> w21
    frame #0 {
      n752 = call "mDrive Send Command.vi"("error in (no error)"=w1616, "Extra"="P", "Command"=T1."Print Parameter", "VISA resource name"=w1618) -> ("error out"=w1615:errorcluster, "read buffer"=w1622:string, "VISA resource name out"=w1617:refnum<visa-resource-name>)  [unwired: 3 in]
      n753 = call "Time Delay33"("error in (no error)"=w1615) -> ("error out"=w1612:errorcluster)  [unwired: 10 in]
      n754 = call "mDrive Send Command.vi"("error in (no error)"=w1612, "Command"=T1."Stop", "VISA resource name"=w1617) -> ("error out"=w1624:errorcluster, "VISA resource name out"=w1625:refnum<visa-resource-name>)  [unwired: 4 in, 1 out]
      n755 = Decimal String To Number(string=w1622, offset=0) -> (number=w1614:i32)  [unwired: 1 in, 1 out]
      n756 = To Long Integer(number=w1614) -> (32bit integer=w1613:i32)
      n757 = VISA Close(VISA resource name=w1625, error in (no error)=w1624) -> ()  [unwired: 1 out]
    }
  }
  n758 = flat-sequence {
    tunnel: w24 -> [w1631]
    tunnel: w23 -> [w1630]
    tunnel: w22 -> [w1629]
    tunnel: w21 -> [w1628]
    frame #0 {
      n759 = Build Array(w1631, w1630, w1629, w1628) -> (w1626:i32[])
      n760 = call-poly <vilib>:"Write To Spreadsheet File.vi"("1D data"=w1626, "file path (dialog if empty)"=path "S:/SSE/IMS/POS.TXT") -> ()  [unwired: 6 in, 1 out]
    }
    frame #1 {
      n761 = property on="Presets" class="Arr (strict)"() -> ("Value"=w1638:i32[][])  [unwired: 2 in, 2 out]
      n762 = property on="Preset positions" class="Ring (strict)"() -> ("Strings []"=w1634:string[])  [unwired: 2 in, 2 out]
      n763 = Number To Decimal String(number=w1638) -> (decimal integer string=w1632:string[][])  [unwired: 1 in]
      n764 = Transpose 2D Array(2D array=w1632) -> (transposed array=w1633:string[][])
      n765 = Build Array (concatenate)(w1634, w1633) -> (w1635:string[][])
      n766 = Transpose 2D Array(2D array=w1635) -> (transposed array=w1636:string[][])
      n767 = call-poly <vilib>:"Write To Spreadsheet File.vi"("2D data"=w1636, "file path (dialog if empty)"=path "S:/SSE/IMS/PRESET.TXT") -> ()  [unwired: 6 in, 1 out]
    }
  }
